vi "Laser handler.vi"(8 "error in (no error)":errorcluster, 11 "Message Queues out":T1) -> (0 "error out":errorcluster, 3 "Message Queue":refnum<queue>)   [LabVIEW 2014]
uses:
  support/Message Queue/All Message Queues.ctl
  support/Message Queue/Message Cluster.ctl
  Engine/Message.ctl
  Teszt/Teszt.ctl
  Teszt/Command.ctl
  Keyence data cluster.ctl
  Keyence Status.ctl
  support/Message Queue/Enqueue Message (Single).vi
  <vilib>/Utility/error.llb/Error Cluster From Error Code.vi
  <vilib>/ErrorRing/Error Ring.xnode
  support/Message Queue/Message Queue.lvlib
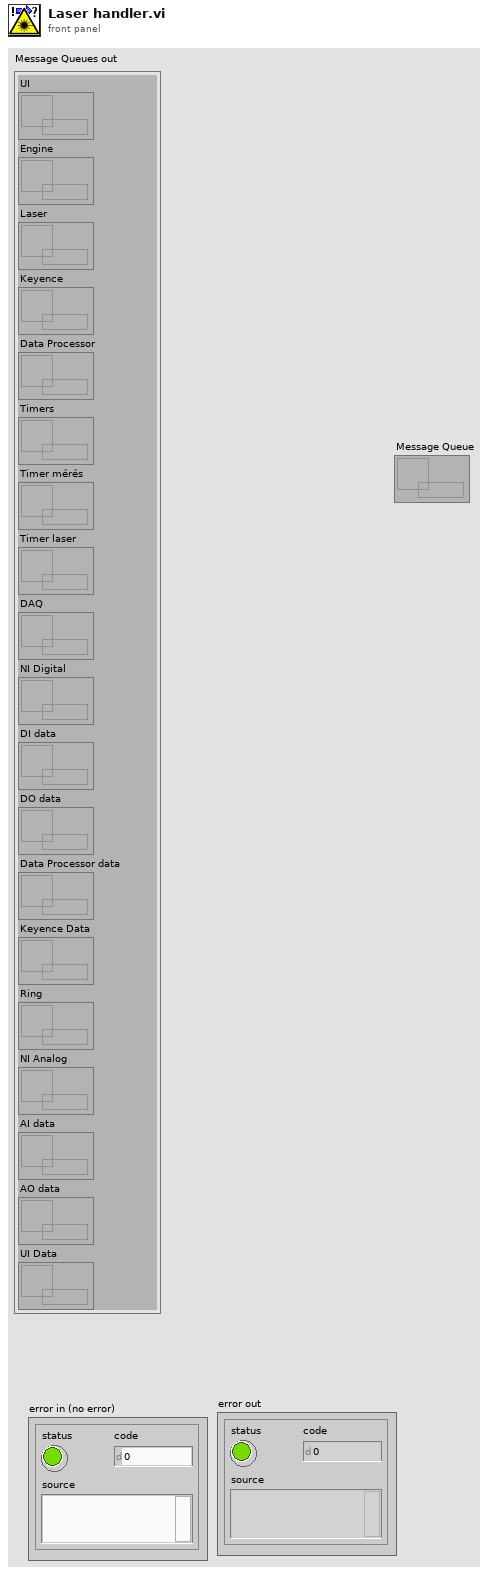
[diagram p1: front panel]
types:
  T1 = typedef "Message Queue.lvlib/All Message Queues.ctl" = cluster{"UI":refnum<queue>, "Engine":refnum<queue>, "Laser":refnum<queue>, "Keyence":refnum<queue>, "Data Processor":refnum<queue>, "Timers":refnum<queue>, "Timer mérés":refnum<queue>, "Timer laser":refnum<queue>, "DAQ":refnum<queue>, "NI Digital":refnum<queue>, "DI data":refnum<queue>, "DO data":refnum<queue>, "Data Processor data":refnum<queue>, "Keyence Data":refnum<queue>, "Ring":refnum<queue>, "NI Analog":refnum<queue>, "AI data":refnum<queue>, "AO data":refnum<queue>, "UI Data":refnum<queue>}
  T2 = typedef "Teszt.ctl" = cluster{"Thread ID":dbl, "Mérésszám":string, "Mérés/Utasítás":string, "Command":T3, "Min":string, "Max":string, "Aktív?":bool, "Log?":bool, "Kiértékelés":bool, "Etalon 1 exp":bool, "Etalon 2 exp":bool, "Etalon 3 exp":bool, "Etalon 4 exp":bool, "Etalon 5 exp":bool}
  T3 = typedef "Command.ctl" = cluster{"Parancs":string, "Paraméter 1":string, "Paraméter 2":string, "Paraméter 3":string, "Paraméter 4":string, "Paraméter 5":string, "Eredmény":string}
  T4 = typedef "Message.ctl" = cluster{"Thread ID":u16, "Callback":string, "Data":variant, "Error":errorcluster}
  T5 = typedef "Keyence data cluster.ctl" = cluster{"Communication Opened":bool, "Status":T6, "IP Address":string, "Laser Disabled":bool}
  T6 = typedef "Keyence Status.ctl" = cluster{"Ready":bool, "Error":bool, "Warning":bool, "Shutter":bool, "Mark Check OK":bool, "Mark Check NG":bool, "Marking Busy":bool, "Program No":u16, "Marking Check Busy":bool, "Marking Completed":bool, "Marking Score":u16, "Marking Error":bool, "Marking Stop":bool, "Program is changing":bool, "Date/Time":timestamp}
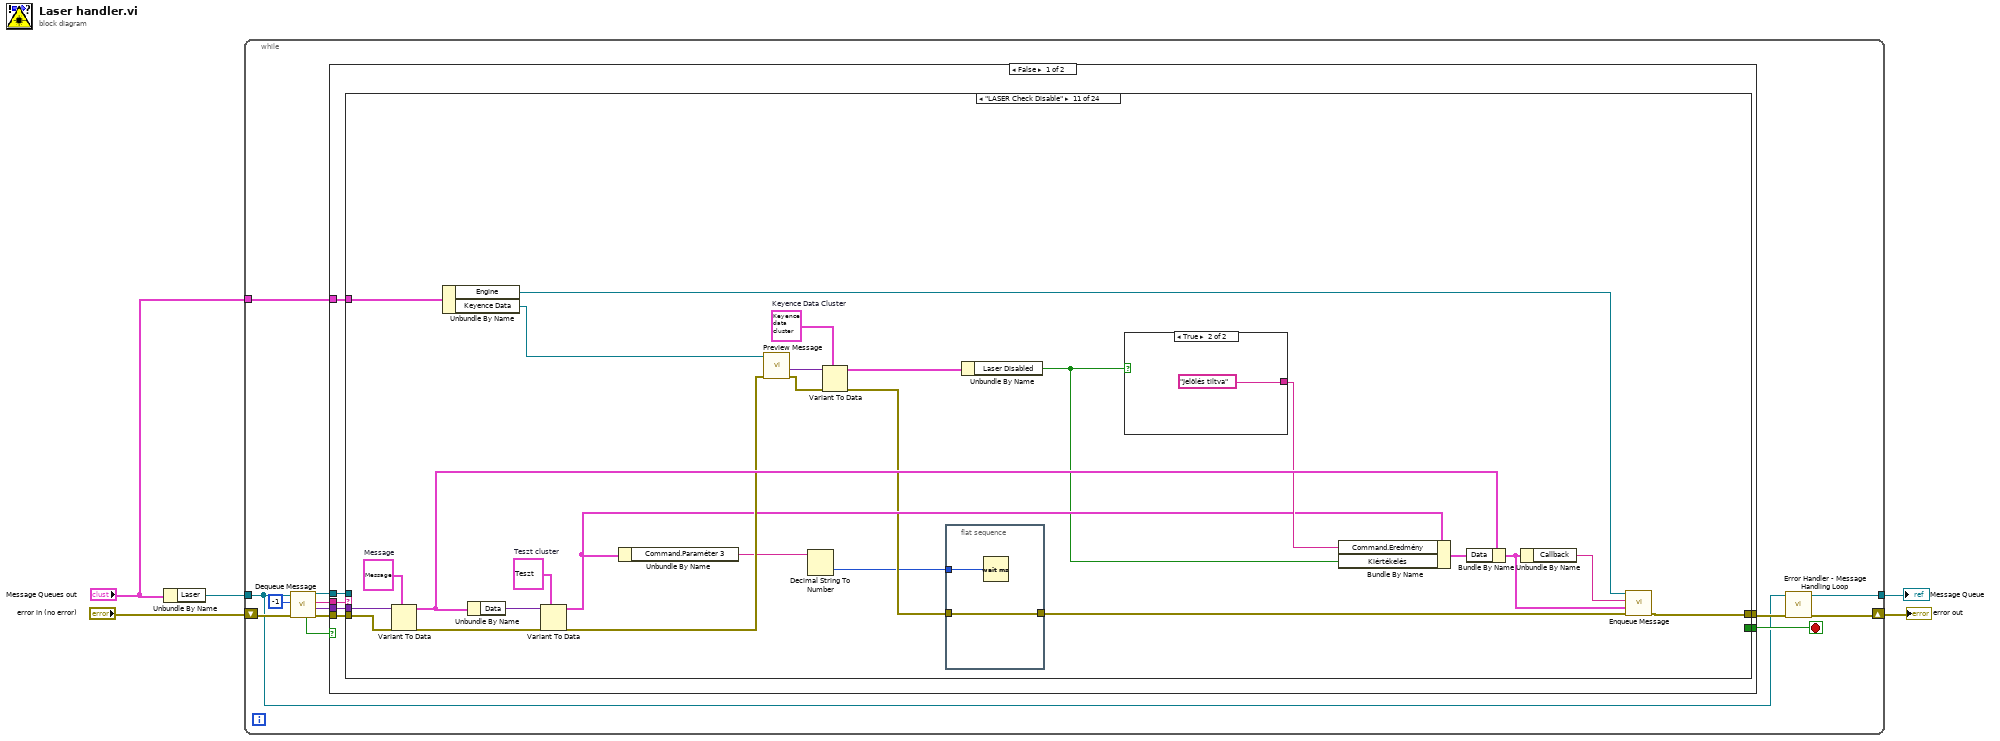
[diagram p0: block diagram]
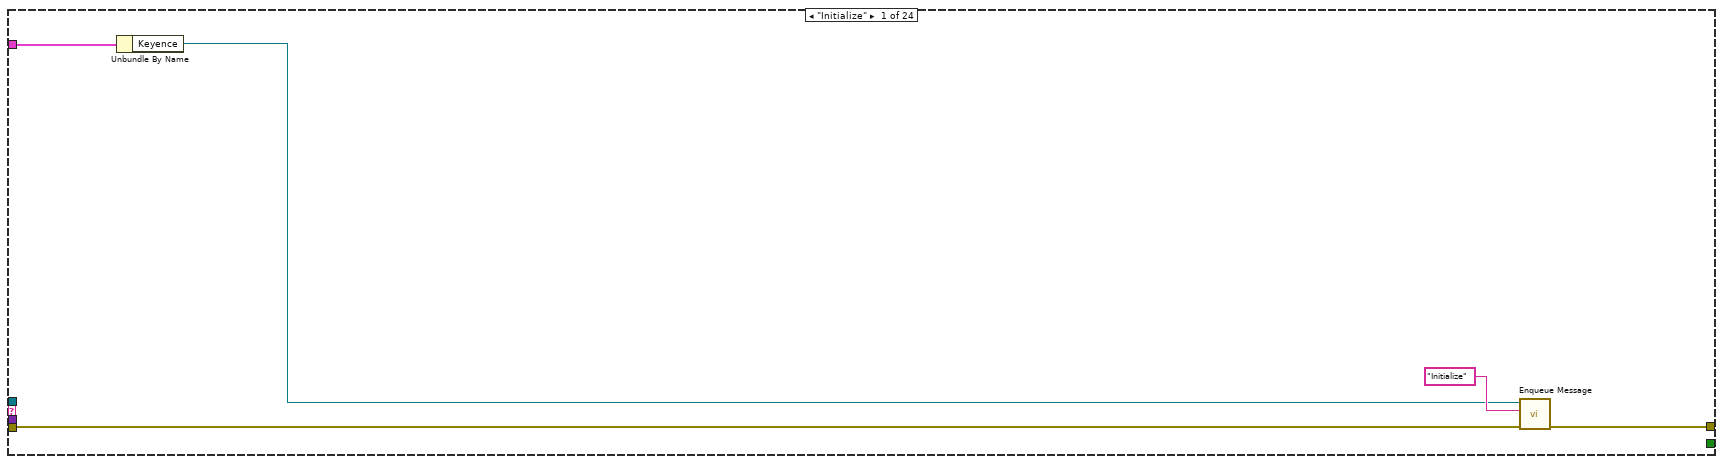
[diagram p2: hidden frame]
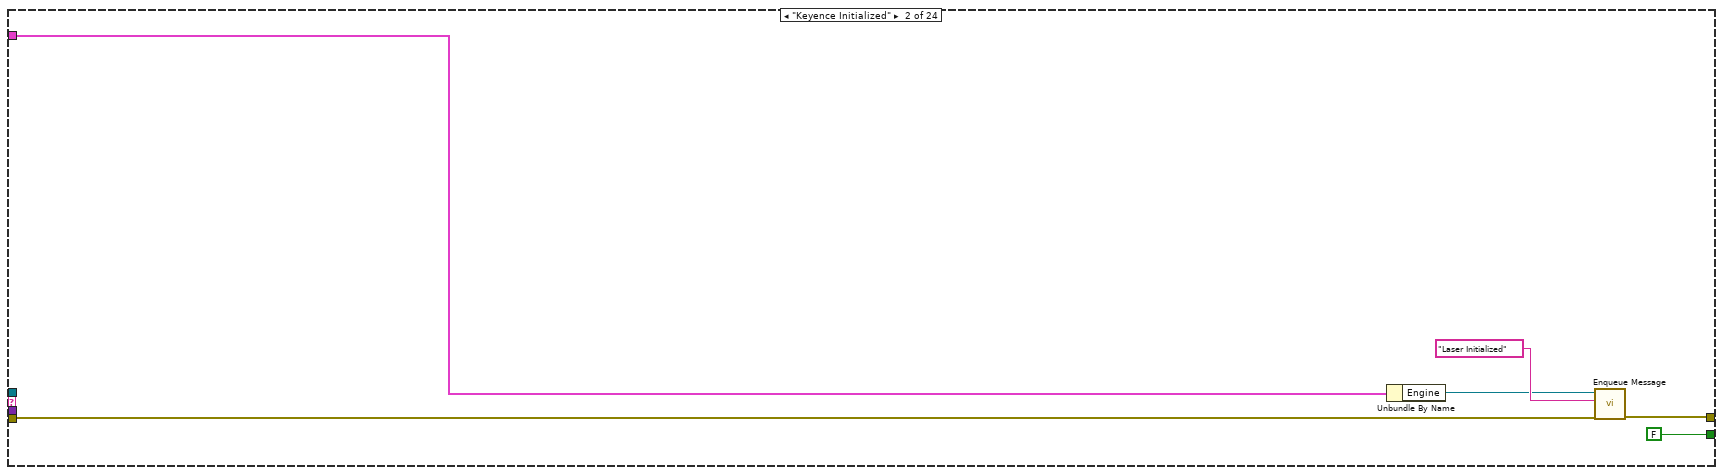
[diagram p3: hidden frame]
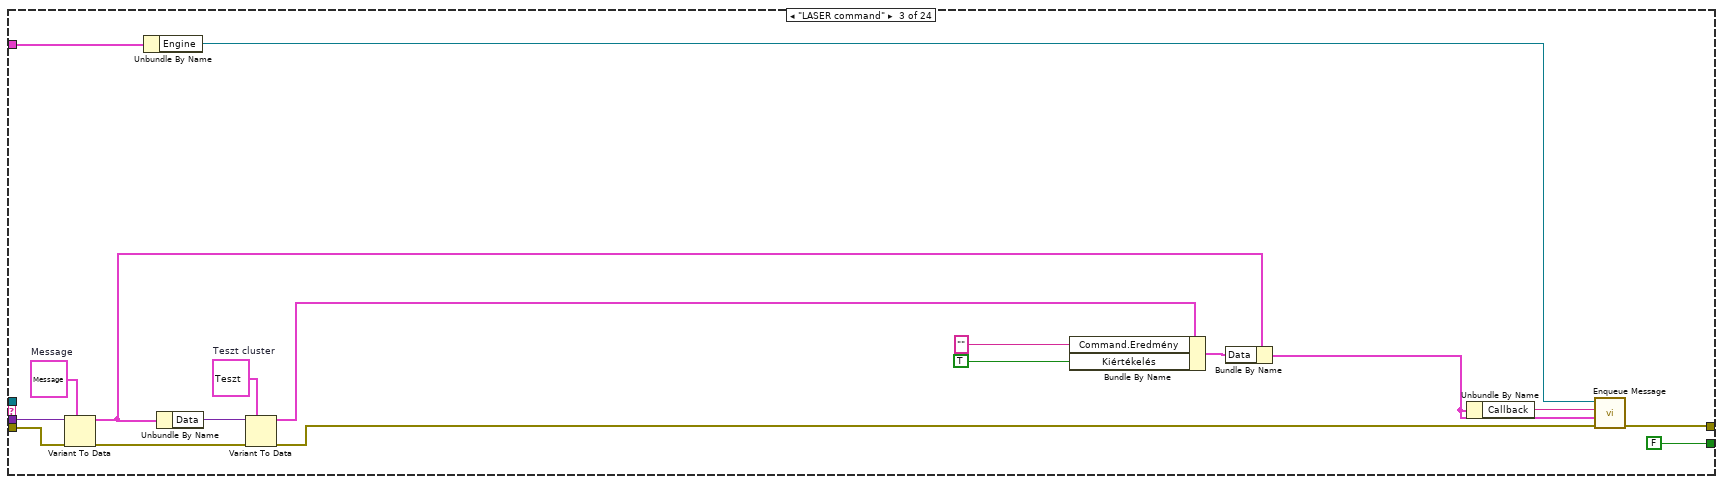
[diagram p4: hidden frame]
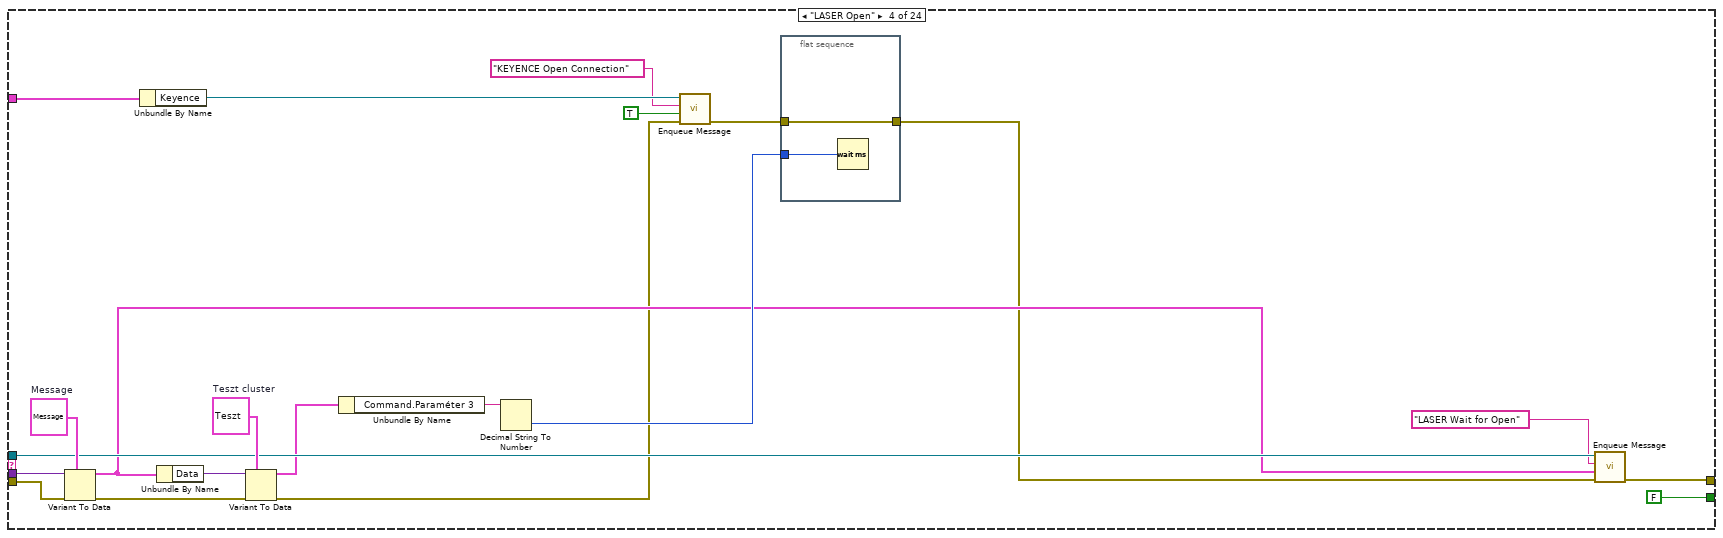
[diagram p5: hidden frame]
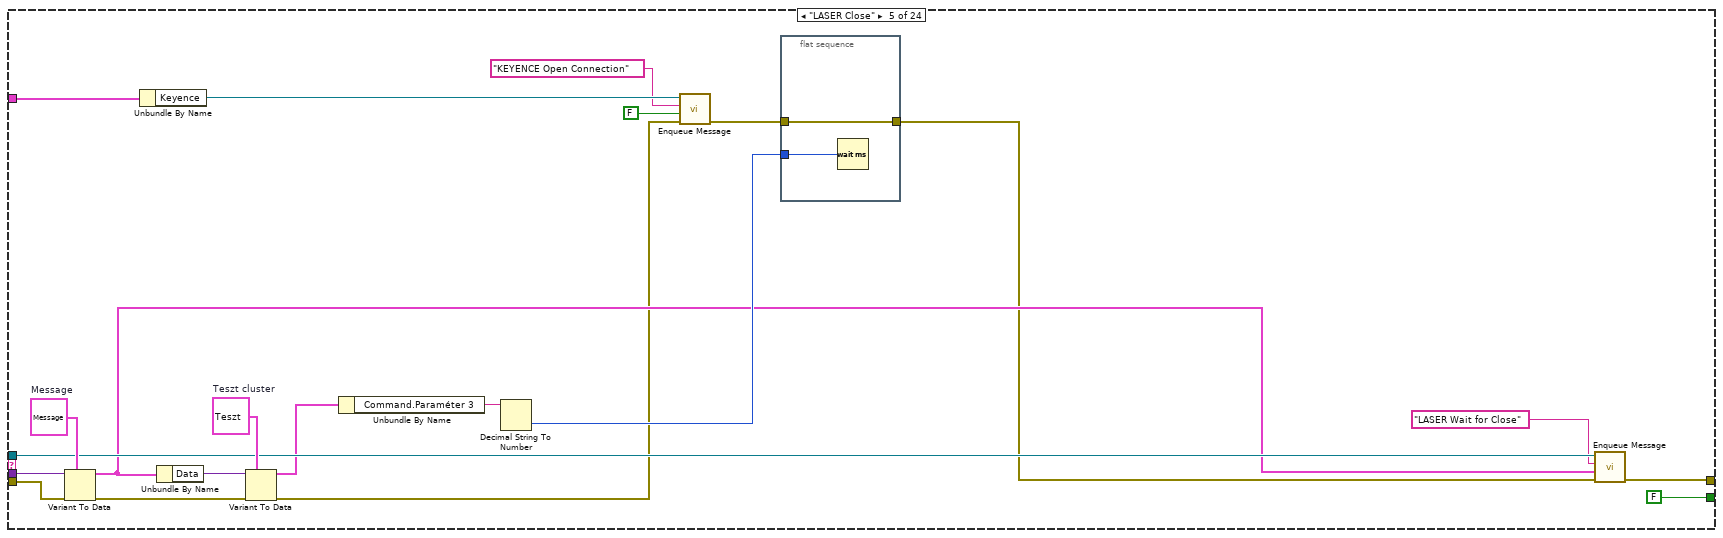
[diagram p6: hidden frame]
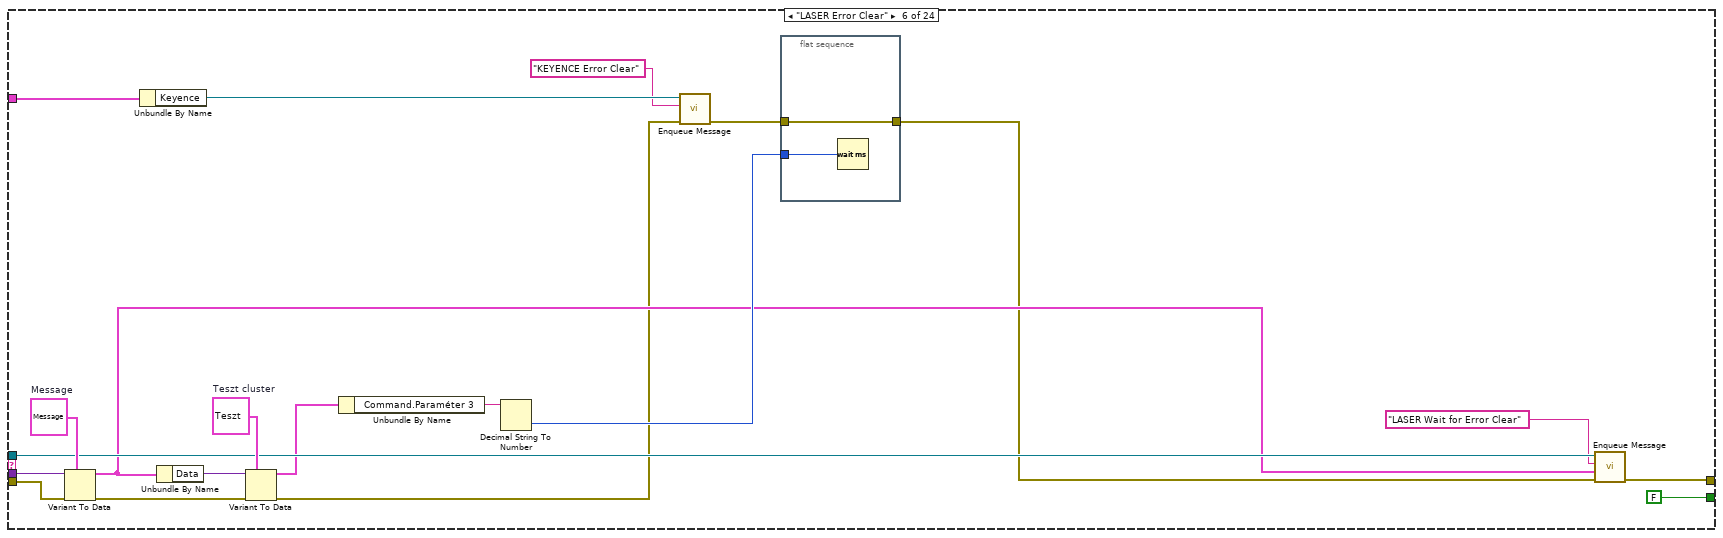
[diagram p7: hidden frame]
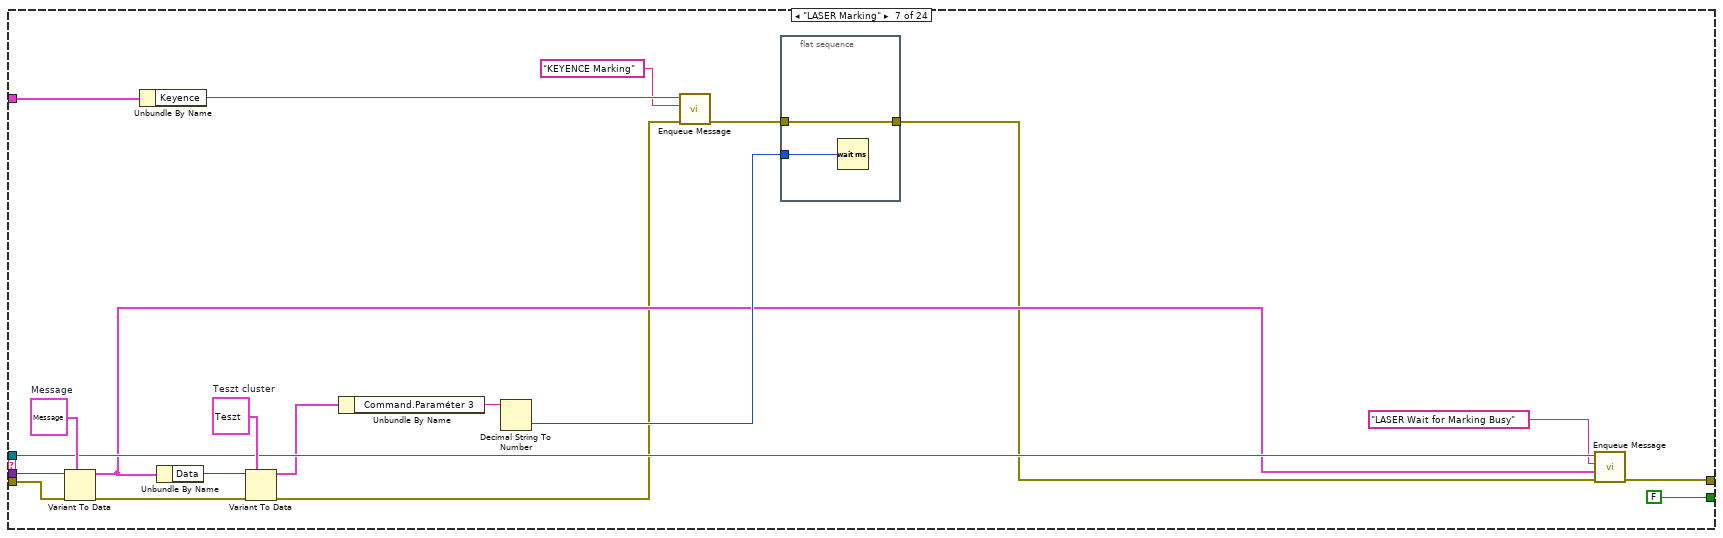
[diagram p8: hidden frame]
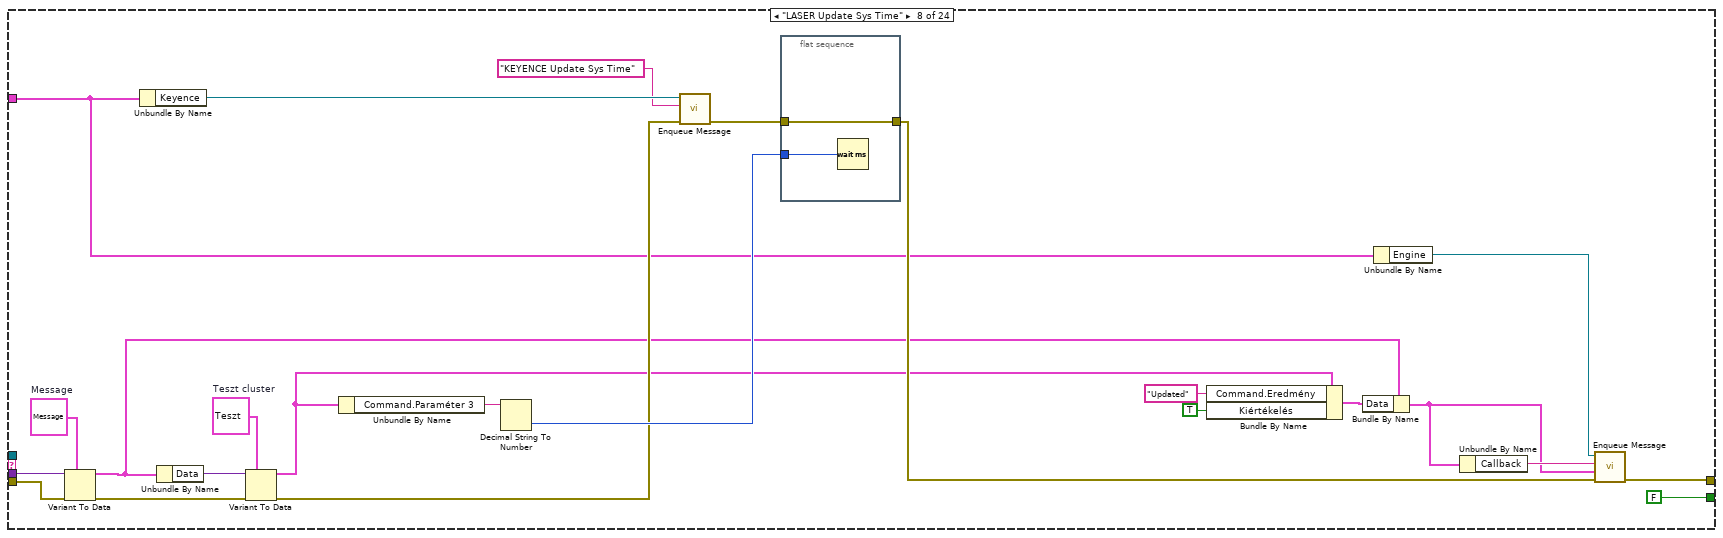
[diagram p9: hidden frame]
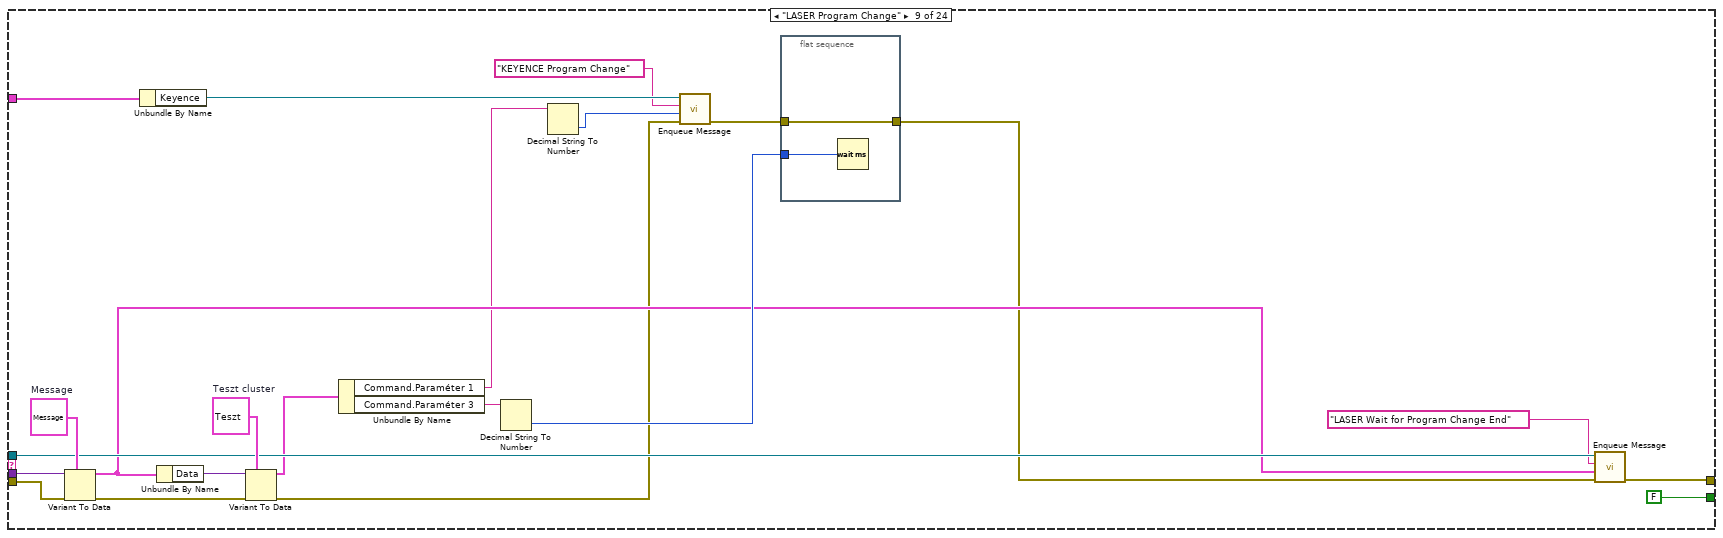
[diagram p10: hidden frame]
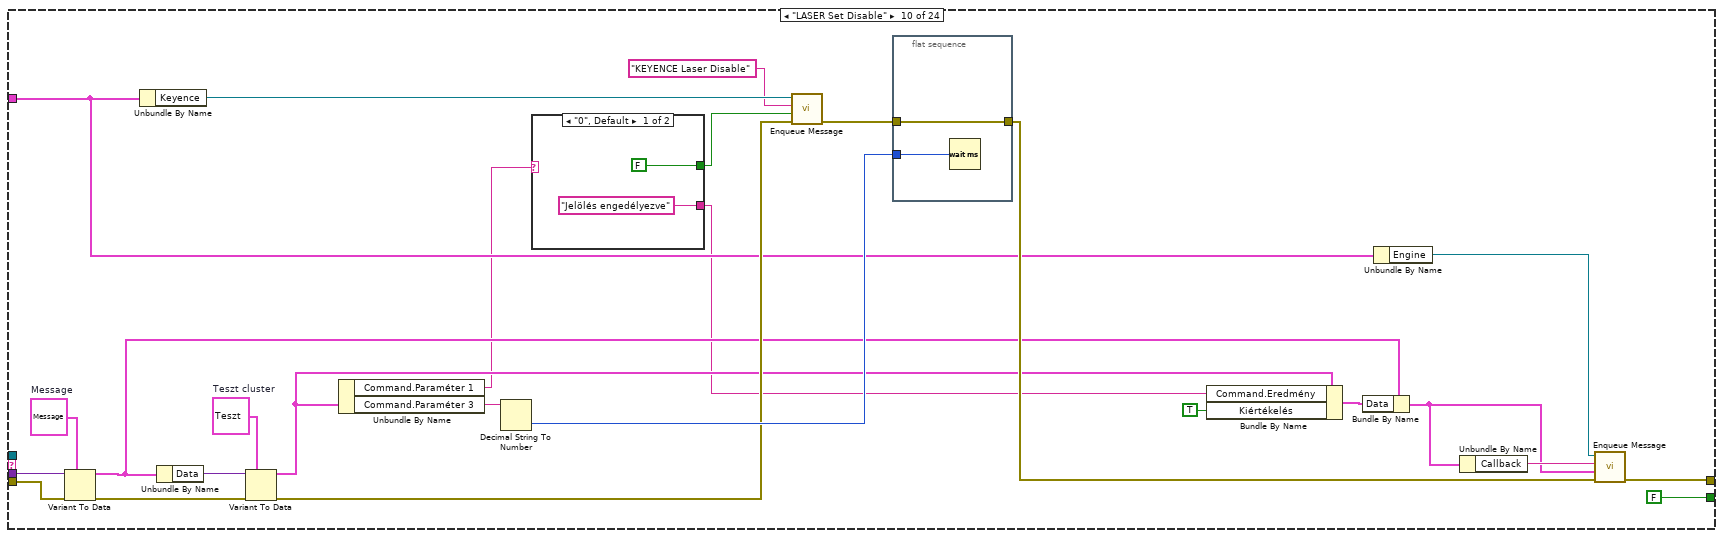
[diagram p11: hidden frame]
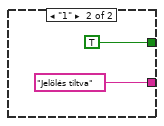
[diagram p12: hidden frame]
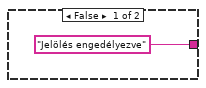
[diagram p13: hidden frame]
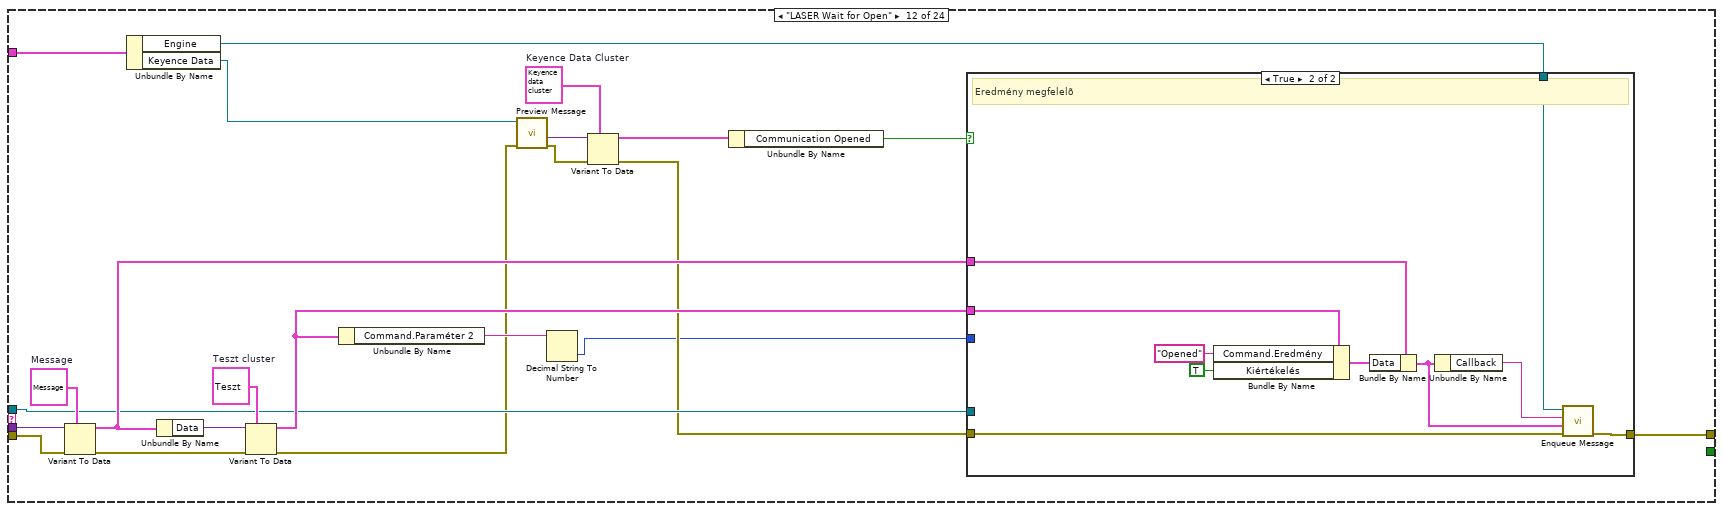
[diagram p14: hidden frame]
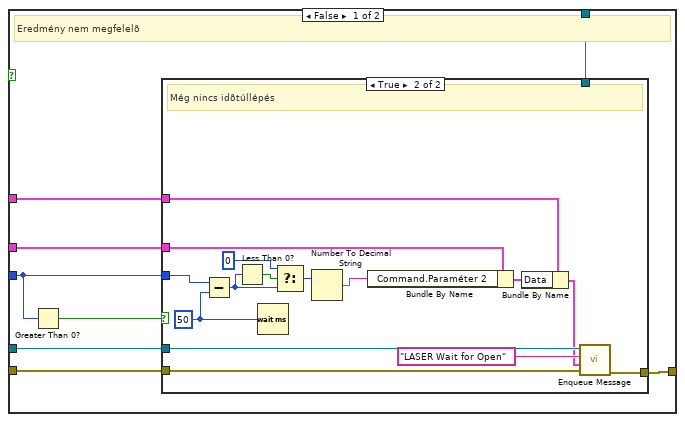
[diagram p15: hidden frame]
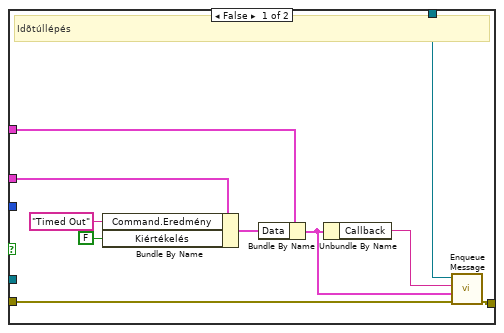
[diagram p16: hidden frame]
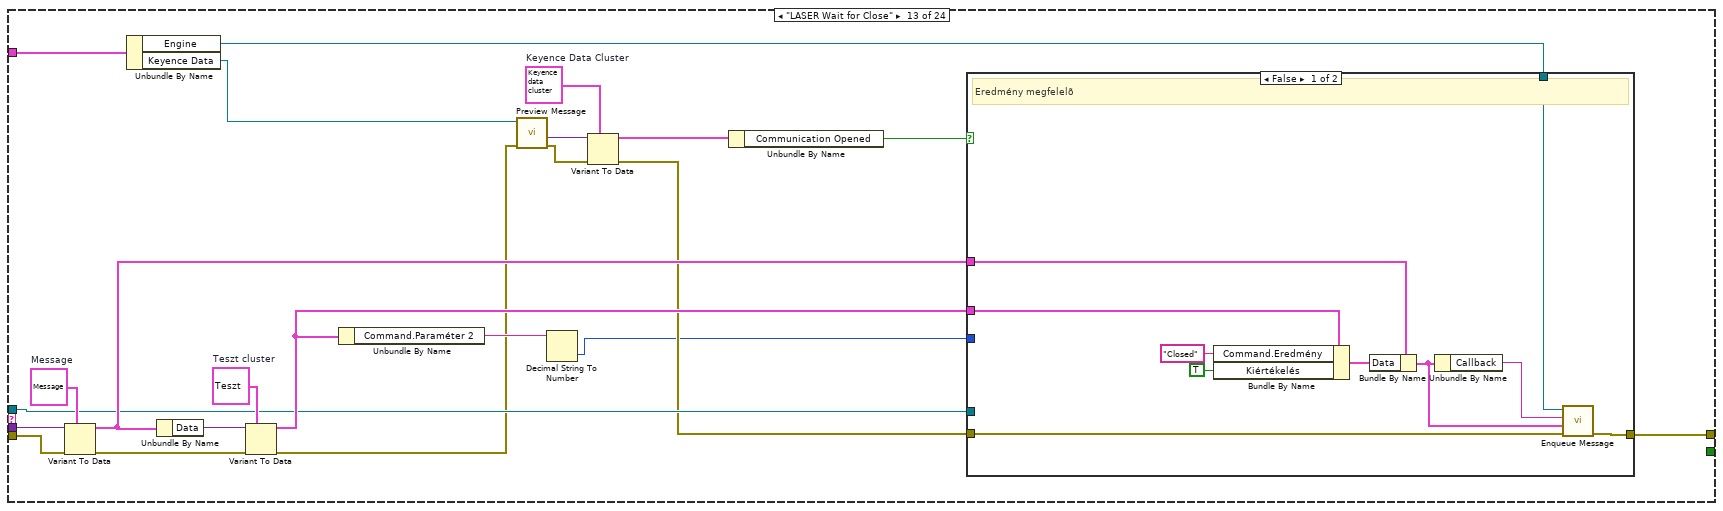
[diagram p17: hidden frame]
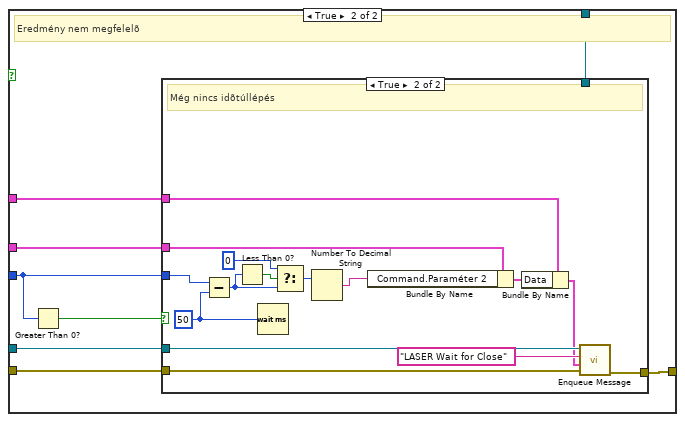
[diagram p18: hidden frame]
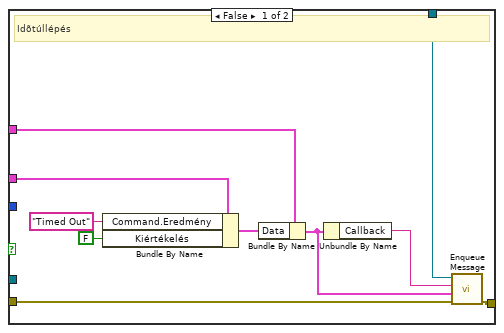
[diagram p19: hidden frame]
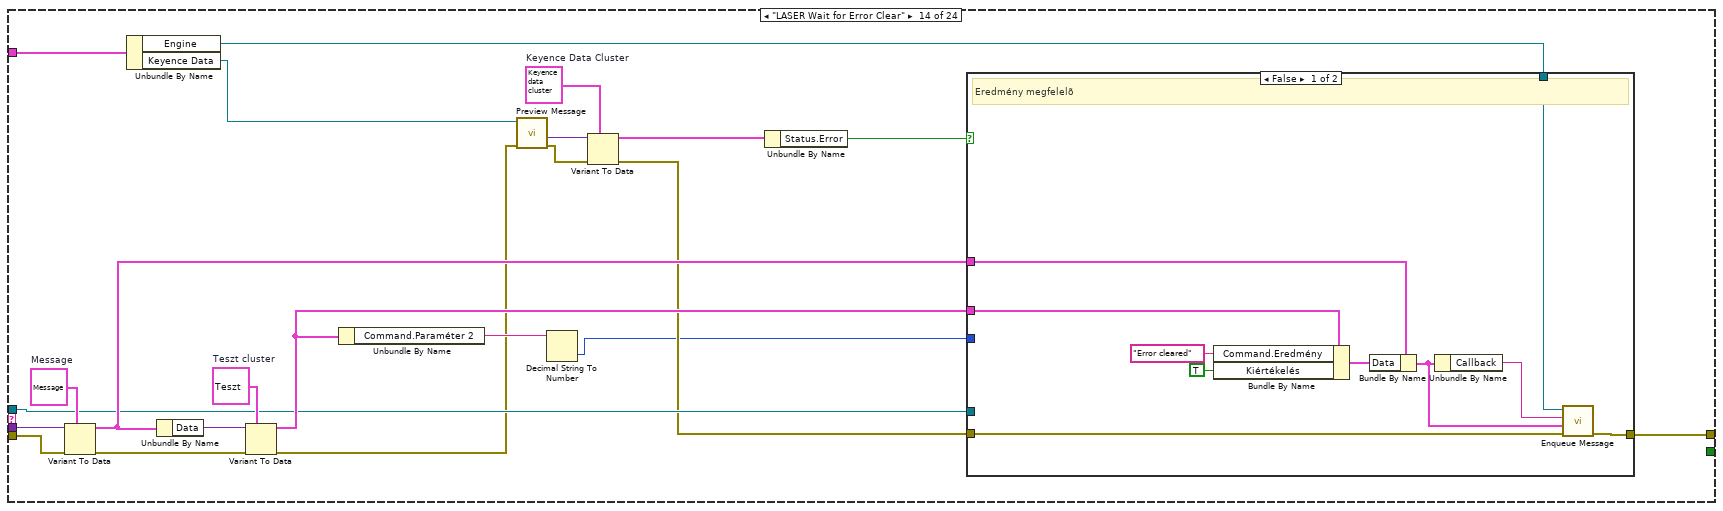
[diagram p20: hidden frame]
diagram:
  n1 = Unbundle By Name("Message Queues out") -> ("Laser"=w2:refnum<queue>)
  n2 = while {
    tunnel: w2 -> [w6]
    shift-right: [w10] -> w5
    shift-left: "error in (no error)" -> [w18]
    tunnel: "Message Queues out" -> [w8]
    tunnel: [w7] -> w1
    stop <- w14 stop-if-true
    n3 = call "Dequeue Message.vi"("error in (no error)"=w18, "timeout in ms (-1)"=-1, "Message Queue"=w6) -> ("error out"=w16:errorcluster, "Message Data"=w11:variant, "Message"=w17:string, "dup Message Queue"=w15:refnum<queue>, "timed out?"=w12:bool)  [unwired: 4 in]
    n4 = case shown="False" w12 {
      tunnel: w17 -> [w25 _]
      tunnel: w16 -> [w24 w804]
      tunnel: w15 -> [w23 _]
      tunnel: [w22 FALSE] -> w14
      tunnel: [w21 w804] -> w9
      tunnel: w11 -> [w20 _]
      tunnel: w8 -> [w19 _]
      frame False {
        n5 = case shown="\"LASER Check Disable\"" w25 {
          selector: w25 -> [_ _ _ _ _ _ _ _ _ _ _ _ _ _ _ _ _ _ _ _ _ _ _ w794]
          tunnel: w24 -> [w28 w31 w46 w68 w91 w113 w135 w163 w185 w215 w245 w271 w336 w401 w466 w529 w589 w651 w720 w773 w774 w788 w791 _]
          tunnel: w23 -> [_ _ _ w66 w89 w111 w133 _ w183 _ _ w265 w330 w395 w460 w523 w583 w645 w714 w772 w777 w787 w793 _]
          tunnel: [w29 w35 w53 w74 w97 w119 w141 w167 w191 w219 w252 w278 w343 w408 w473 w536 w596 w658 w727 w771 w778 w789 w790 w795] -> w21
          tunnel: [_ FALSE FALSE FALSE FALSE FALSE FALSE FALSE FALSE FALSE _ _ _ _ _ _ _ _ _ _ _ _ TRUE FALSE] -> w22
          tunnel: w20 -> [_ _ w45 w67 w90 w112 w134 w162 w184 w214 w244 w270 w335 w400 w465 w528 w588 w650 w719 _ w775 _ _ _]
          tunnel: w19 -> [w27 w32 w51 w73 w96 w118 w140 w146 w190 w199 w250 w276 w341 w406 w471 w534 w594 w656 w725 _ w776 _ _ _]
          frame "Initialize" {
            n6 = Unbundle By Name(w27) -> ("Keyence"=w26:refnum<queue>)
            n7 = call-poly "Enqueue Message.vi"("error in (no error)"=w28, "Message"="Initialize", "Message Queue"=w26) -> ("error out"=w29:errorcluster)  [unwired: 7 in, 1 out]
          }
          frame "Keyence Initialized" {
            n8 = Unbundle By Name(w32) -> ("Engine"=w33:refnum<queue>)
            n9 = call-poly "Enqueue Message.vi"("error in (no error)"=w31, "Message"="Laser Initialized", "Message Queue"=w33) -> ("error out"=w35:errorcluster)  [unwired: 7 in, 1 out]
          }
          frame "LASER command" {
            w47 = T2 {"Thread ID"=0.0, "Mérésszám"="", "Mérés/Utasítás"="", "Command"={"Parancs"="", "Paraméter 1"="", "Paraméter 2"="", "Paraméter 3"="", "Paraméter 4"="", "Paraméter 5"="", "Eredmény"=""}, "Min"="", "Max"="", "Aktív?"=FALSE, "Log?"=FALSE, "Kiértékelés"=FALSE, "Etalon 1 exp"=FALSE, "Etalon 2 exp"=FALSE, "Etalon 3 exp"=FALSE, "Etalon 4 exp"=FALSE, "Etalon 5 exp"=FALSE}  # Teszt cluster
            w50 = T4 {"Thread ID"=0, "Callback"="", "Data"=variant, "Error"={"status"=FALSE, "code"=0, "source"=""}}  # Message
            n10 = Variant To Data(error in=w46, type=w50, Variant=w45) -> (data=w41:T4, error out=w49:errorcluster)
            n11 = Unbundle By Name(w51) -> ("Engine"=w52:refnum<queue>)
            n12 = Unbundle By Name(w41) -> ("Data"=w48:variant)
            n13 = Variant To Data(error in=w49, type=w47, Variant=w48) -> (data=w37:T2, error out=w40:errorcluster)
            n14 = Bundle By Name(cluster=w37, "Command.Eredmény"="", "Kiértékelés"=TRUE) -> (w44:T2)
            n15 = Bundle By Name(cluster=w41, "Data"=w44) -> (w42:T4)
            n16 = Unbundle By Name(w42) -> ("Callback"=w43:string)
            n17 = call-poly "Enqueue Message.vi"("error in (no error)"=w40, "Message Data"=w42, "Message"=w43, "Message Queue"=w52) -> ("error out"=w53:errorcluster)  [unwired: 6 in, 1 out]
          }
          frame "LASER Open" {
            w69 = T2 {"Thread ID"=0.0, "Mérésszám"="", "Mérés/Utasítás"="", "Command"={"Parancs"="", "Paraméter 1"="", "Paraméter 2"="", "Paraméter 3"="", "Paraméter 4"="", "Paraméter 5"="", "Eredmény"=""}, "Min"="", "Max"="", "Aktív?"=FALSE, "Log?"=FALSE, "Kiértékelés"=FALSE, "Etalon 1 exp"=FALSE, "Etalon 2 exp"=FALSE, "Etalon 3 exp"=FALSE, "Etalon 4 exp"=FALSE, "Etalon 5 exp"=FALSE}  # Teszt cluster
            w72 = T4 {"Thread ID"=0, "Callback"="", "Data"=variant, "Error"={"status"=FALSE, "code"=0, "source"=""}}  # Message
            n18 = Variant To Data(error in=w68, type=w72, Variant=w67) -> (data=w58:T4, error out=w71:errorcluster)
            n19 = Unbundle By Name(w73) -> ("Keyence"=w64:refnum<queue>)
            n20 = Unbundle By Name(w58) -> ("Data"=w70:variant)
            n21 = Variant To Data(error in=w71, type=w69, Variant=w70) -> (data=w61:T2, error out=w56:errorcluster)
            n22 = Unbundle By Name(w61) -> ("Command.Paraméter 3"=w60:string)
            n23 = Decimal String To Number(string=w60) -> (number=w59:i32)  [unwired: 2 in, 1 out]
            n24 = call-poly "Enqueue Message.vi"("error in (no error)"=w56, "Message Data"=TRUE, "Message"="KEYENCE Open Connection", "Message Queue"=w64) -> ("error out"=w57:errorcluster)  [unwired: 6 in, 1 out]
            n25 = flat-sequence {
              tunnel: w59 -> [w77]
              tunnel: w57 -> [w76]
              tunnel: [w76] -> w55
              frame #0 {
                n26 = Wait (ms)(milliseconds to wait=w77) -> ()  [unwired: 1 out]
              }
            }
            n27 = call-poly "Enqueue Message.vi"("error in (no error)"=w55, "Message Data"=w58, "Message"="LASER Wait for Open", "Message Queue"=w66) -> ("error out"=w74:errorcluster)  [unwired: 6 in, 1 out]
          }
          frame "LASER Close" {
            w92 = T2 {"Thread ID"=0.0, "Mérésszám"="", "Mérés/Utasítás"="", "Command"={"Parancs"="", "Paraméter 1"="", "Paraméter 2"="", "Paraméter 3"="", "Paraméter 4"="", "Paraméter 5"="", "Eredmény"=""}, "Min"="", "Max"="", "Aktív?"=FALSE, "Log?"=FALSE, "Kiértékelés"=FALSE, "Etalon 1 exp"=FALSE, "Etalon 2 exp"=FALSE, "Etalon 3 exp"=FALSE, "Etalon 4 exp"=FALSE, "Etalon 5 exp"=FALSE}  # Teszt cluster
            w95 = T4 {"Thread ID"=0, "Callback"="", "Data"=variant, "Error"={"status"=FALSE, "code"=0, "source"=""}}  # Message
            n28 = Variant To Data(error in=w91, type=w95, Variant=w90) -> (data=w81:T4, error out=w94:errorcluster)
            n29 = Unbundle By Name(w96) -> ("Keyence"=w87:refnum<queue>)
            n30 = Unbundle By Name(w81) -> ("Data"=w93:variant)
            n31 = Variant To Data(error in=w94, type=w92, Variant=w93) -> (data=w84:T2, error out=w79:errorcluster)
            n32 = Unbundle By Name(w84) -> ("Command.Paraméter 3"=w83:string)
            n33 = Decimal String To Number(string=w83) -> (number=w82:i32)  [unwired: 2 in, 1 out]
            n34 = call-poly "Enqueue Message.vi"("error in (no error)"=w79, "Message Data"=FALSE, "Message"="KEYENCE Open Connection", "Message Queue"=w87) -> ("error out"=w80:errorcluster)  [unwired: 6 in, 1 out]
            n35 = flat-sequence {
              tunnel: w82 -> [w100]
              tunnel: w80 -> [w99]
              tunnel: [w99] -> w78
              frame #0 {
                n36 = Wait (ms)(milliseconds to wait=w100) -> ()  [unwired: 1 out]
              }
            }
            n37 = call-poly "Enqueue Message.vi"("error in (no error)"=w78, "Message Data"=w81, "Message"="LASER Wait for Close", "Message Queue"=w89) -> ("error out"=w97:errorcluster)  [unwired: 6 in, 1 out]
          }
          frame "LASER Error Clear" {
            w114 = T2 {"Thread ID"=0.0, "Mérésszám"="", "Mérés/Utasítás"="", "Command"={"Parancs"="", "Paraméter 1"="", "Paraméter 2"="", "Paraméter 3"="", "Paraméter 4"="", "Paraméter 5"="", "Eredmény"=""}, "Min"="", "Max"="", "Aktív?"=FALSE, "Log?"=FALSE, "Kiértékelés"=FALSE, "Etalon 1 exp"=FALSE, "Etalon 2 exp"=FALSE, "Etalon 3 exp"=FALSE, "Etalon 4 exp"=FALSE, "Etalon 5 exp"=FALSE}  # Teszt cluster
            w117 = T4 {"Thread ID"=0, "Callback"="", "Data"=variant, "Error"={"status"=FALSE, "code"=0, "source"=""}}  # Message
            n38 = Variant To Data(error in=w113, type=w117, Variant=w112) -> (data=w104:T4, error out=w116:errorcluster)
            n39 = Unbundle By Name(w118) -> ("Keyence"=w109:refnum<queue>)
            n40 = Unbundle By Name(w104) -> ("Data"=w115:variant)
            n41 = Variant To Data(error in=w116, type=w114, Variant=w115) -> (data=w107:T2, error out=w102:errorcluster)
            n42 = Unbundle By Name(w107) -> ("Command.Paraméter 3"=w106:string)
            n43 = Decimal String To Number(string=w106) -> (number=w105:i32)  [unwired: 2 in, 1 out]
            n44 = call-poly "Enqueue Message.vi"("error in (no error)"=w102, "Message"="KEYENCE Error Clear", "Message Queue"=w109) -> ("error out"=w103:errorcluster)  [unwired: 7 in, 1 out]
            n45 = flat-sequence {
              tunnel: w105 -> [w122]
              tunnel: w103 -> [w121]
              tunnel: [w121] -> w101
              frame #0 {
                n46 = Wait (ms)(milliseconds to wait=w122) -> ()  [unwired: 1 out]
              }
            }
            n47 = call-poly "Enqueue Message.vi"("error in (no error)"=w101, "Message Data"=w104, "Message"="LASER Wait for Error Clear", "Message Queue"=w111) -> ("error out"=w119:errorcluster)  [unwired: 6 in, 1 out]
          }
          frame "LASER Marking" {
            w136 = T2 {"Thread ID"=0.0, "Mérésszám"="", "Mérés/Utasítás"="", "Command"={"Parancs"="", "Paraméter 1"="", "Paraméter 2"="", "Paraméter 3"="", "Paraméter 4"="", "Paraméter 5"="", "Eredmény"=""}, "Min"="", "Max"="", "Aktív?"=FALSE, "Log?"=FALSE, "Kiértékelés"=FALSE, "Etalon 1 exp"=FALSE, "Etalon 2 exp"=FALSE, "Etalon 3 exp"=FALSE, "Etalon 4 exp"=FALSE, "Etalon 5 exp"=FALSE}  # Teszt cluster
            w139 = T4 {"Thread ID"=0, "Callback"="", "Data"=variant, "Error"={"status"=FALSE, "code"=0, "source"=""}}  # Message
            n48 = Variant To Data(error in=w135, type=w139, Variant=w134) -> (data=w126:T4, error out=w138:errorcluster)
            n49 = Unbundle By Name(w140) -> ("Keyence"=w131:refnum<queue>)
            n50 = Unbundle By Name(w126) -> ("Data"=w137:variant)
            n51 = Variant To Data(error in=w138, type=w136, Variant=w137) -> (data=w129:T2, error out=w124:errorcluster)
            n52 = Unbundle By Name(w129) -> ("Command.Paraméter 3"=w128:string)
            n53 = Decimal String To Number(string=w128) -> (number=w127:i32)  [unwired: 2 in, 1 out]
            n54 = call-poly "Enqueue Message.vi"("error in (no error)"=w124, "Message"="KEYENCE Marking", "Message Queue"=w131) -> ("error out"=w125:errorcluster)  [unwired: 7 in, 1 out]
            n55 = flat-sequence {
              tunnel: w127 -> [w144]
              tunnel: w125 -> [w143]
              tunnel: [w143] -> w123
              frame #0 {
                n56 = Wait (ms)(milliseconds to wait=w144) -> ()  [unwired: 1 out]
              }
            }
            n57 = call-poly "Enqueue Message.vi"("error in (no error)"=w123, "Message Data"=w126, "Message"="LASER Wait for Marking Busy", "Message Queue"=w133) -> ("error out"=w141:errorcluster)  [unwired: 6 in, 1 out]
          }
          frame "LASER Update Sys Time" {
            w164 = T2 {"Thread ID"=0.0, "Mérésszám"="", "Mérés/Utasítás"="", "Command"={"Parancs"="", "Paraméter 1"="", "Paraméter 2"="", "Paraméter 3"="", "Paraméter 4"="", "Paraméter 5"="", "Eredmény"=""}, "Min"="", "Max"="", "Aktív?"=FALSE, "Log?"=FALSE, "Kiértékelés"=FALSE, "Etalon 1 exp"=FALSE, "Etalon 2 exp"=FALSE, "Etalon 3 exp"=FALSE, "Etalon 4 exp"=FALSE, "Etalon 5 exp"=FALSE}  # Teszt cluster
            w148 = T4 {"Thread ID"=0, "Callback"="", "Data"=variant, "Error"={"status"=FALSE, "code"=0, "source"=""}}  # Message
            n58 = Variant To Data(error in=w163, type=w148, Variant=w162) -> (data=w147:T4, error out=w166:errorcluster)
            n59 = Unbundle By Name(w146) -> ("Keyence"=w161:refnum<queue>)
            n60 = Unbundle By Name(w147) -> ("Data"=w165:variant)
            n61 = Variant To Data(error in=w166, type=w164, Variant=w165) -> (data=w149:T2, error out=w156:errorcluster)
            n62 = Unbundle By Name(w149) -> ("Command.Paraméter 3"=w159:string)
            n63 = Decimal String To Number(string=w159) -> (number=w158:i32)  [unwired: 2 in, 1 out]
            n64 = call-poly "Enqueue Message.vi"("error in (no error)"=w156, "Message"="KEYENCE Update Sys Time", "Message Queue"=w161) -> ("error out"=w157:errorcluster)  [unwired: 7 in, 1 out]
            n65 = flat-sequence {
              tunnel: w158 -> [w170]
              tunnel: w157 -> [w169]
              tunnel: [w169] -> w155
              frame #0 {
                n66 = Wait (ms)(milliseconds to wait=w170) -> ()  [unwired: 1 out]
              }
            }
            n67 = Bundle By Name(cluster=w149, "Command.Eredmény"="Updated", "Kiértékelés"=TRUE) -> (w154:T2)
            n68 = Bundle By Name(cluster=w147, "Data"=w154) -> (w150:T4)
            n69 = Unbundle By Name(w146) -> ("Engine"=w145:refnum<queue>)
            n70 = Unbundle By Name(w150) -> ("Callback"=w151:string)
            n71 = call-poly "Enqueue Message.vi"("error in (no error)"=w155, "Message Data"=w150, "Message"=w151, "Message Queue"=w145) -> ("error out"=w167:errorcluster)  [unwired: 6 in, 1 out]
          }
          frame "LASER Program Change" {
            w186 = T2 {"Thread ID"=0.0, "Mérésszám"="", "Mérés/Utasítás"="", "Command"={"Parancs"="", "Paraméter 1"="", "Paraméter 2"="", "Paraméter 3"="", "Paraméter 4"="", "Paraméter 5"="", "Eredmény"=""}, "Min"="", "Max"="", "Aktív?"=FALSE, "Log?"=FALSE, "Kiértékelés"=FALSE, "Etalon 1 exp"=FALSE, "Etalon 2 exp"=FALSE, "Etalon 3 exp"=FALSE, "Etalon 4 exp"=FALSE, "Etalon 5 exp"=FALSE}  # Teszt cluster
            w189 = T4 {"Thread ID"=0, "Callback"="", "Data"=variant, "Error"={"status"=FALSE, "code"=0, "source"=""}}  # Message
            n72 = Variant To Data(error in=w185, type=w189, Variant=w184) -> (data=w176:T4, error out=w188:errorcluster)
            n73 = Unbundle By Name(w190) -> ("Keyence"=w181:refnum<queue>)
            n74 = Unbundle By Name(w176) -> ("Data"=w187:variant)
            n75 = Variant To Data(error in=w188, type=w186, Variant=w187) -> (data=w179:T2, error out=w174:errorcluster)
            n76 = Unbundle By Name(w179) -> ("Command.Paraméter 1"=w172:string, "Command.Paraméter 3"=w178:string)
            n77 = Decimal String To Number(string=w178) -> (number=w177:i32)  [unwired: 2 in, 1 out]
            n78 = Decimal String To Number(string=w172) -> (number=w171:i32)  [unwired: 2 in, 1 out]
            n79 = call-poly "Enqueue Message.vi"("error in (no error)"=w174, "Message Data"=w171, "Message"="KEYENCE Program Change", "Message Queue"=w181) -> ("error out"=w175:errorcluster)  [unwired: 6 in, 1 out]
            n80 = flat-sequence {
              tunnel: w177 -> [w194]
              tunnel: w175 -> [w193]
              tunnel: [w193] -> w173
              frame #0 {
                n81 = Wait (ms)(milliseconds to wait=w194) -> ()  [unwired: 1 out]
              }
            }
            n82 = call-poly "Enqueue Message.vi"("error in (no error)"=w173, "Message Data"=w176, "Message"="LASER Wait for Program Change End", "Message Queue"=w183) -> ("error out"=w191:errorcluster)  [unwired: 6 in, 1 out]
          }
          frame "LASER Set Disable" {
            w216 = T2 {"Thread ID"=0.0, "Mérésszám"="", "Mérés/Utasítás"="", "Command"={"Parancs"="", "Paraméter 1"="", "Paraméter 2"="", "Paraméter 3"="", "Paraméter 4"="", "Paraméter 5"="", "Eredmény"=""}, "Min"="", "Max"="", "Aktív?"=FALSE, "Log?"=FALSE, "Kiértékelés"=FALSE, "Etalon 1 exp"=FALSE, "Etalon 2 exp"=FALSE, "Etalon 3 exp"=FALSE, "Etalon 4 exp"=FALSE, "Etalon 5 exp"=FALSE}  # Teszt cluster
            w201 = T4 {"Thread ID"=0, "Callback"="", "Data"=variant, "Error"={"status"=FALSE, "code"=0, "source"=""}}  # Message
            n83 = Variant To Data(error in=w215, type=w201, Variant=w214) -> (data=w200:T4, error out=w218:errorcluster)
            n84 = Unbundle By Name(w199) -> ("Keyence"=w213:refnum<queue>)
            n85 = Unbundle By Name(w200) -> ("Data"=w217:variant)
            n86 = Variant To Data(error in=w218, type=w216, Variant=w217) -> (data=w202:T2, error out=w208:errorcluster)
            n87 = Unbundle By Name(w202) -> ("Command.Paraméter 1"=w196:string, "Command.Paraméter 3"=w211:string)
            n88 = Decimal String To Number(string=w211) -> (number=w210:i32)  [unwired: 2 in, 1 out]
            n89 = case shown="\"0\", Default" w196 {
              tunnel: [FALSE ("Run") TRUE ("Run")] -> w197
              tunnel: ["Jelölés engedélyezve" "Jelölés tiltva"] -> w195
              frame "0", Default {
              }
              frame "1" {
              }
            }
            n90 = call-poly "Enqueue Message.vi"("error in (no error)"=w208, "Message Data"=w197, "Message"="KEYENCE Laser Disable", "Message Queue"=w213) -> ("error out"=w209:errorcluster)  [unwired: 6 in, 1 out]
            n91 = flat-sequence {
              tunnel: w210 -> [w226]
              tunnel: w209 -> [w225]
              tunnel: [w225] -> w207
              frame #0 {
                n92 = Wait (ms)(milliseconds to wait=w226) -> ()  [unwired: 1 out]
              }
            }
            n93 = Bundle By Name(cluster=w202, "Command.Eredmény"=w195, "Kiértékelés"=TRUE) -> (w206:T2)
            n94 = Bundle By Name(cluster=w200, "Data"=w206) -> (w203:T4)
            n95 = Unbundle By Name(w199) -> ("Engine"=w198:refnum<queue>)
            n96 = Unbundle By Name(w203) -> ("Callback"=w204:string)
            n97 = call-poly "Enqueue Message.vi"("error in (no error)"=w207, "Message Data"=w203, "Message"=w204, "Message Queue"=w198) -> ("error out"=w219:errorcluster)  [unwired: 6 in, 1 out]
          }
          frame "LASER Check Disable" {
            w240 = T5 {"Communication Opened"=FALSE, "Status"={"Ready"=FALSE, "Error"=FALSE, "Warning"=FALSE, "Shutter"=FALSE, "Mark Check OK"=FALSE, "Mark Check NG"=FALSE, "Marking Busy"=FALSE, "Program No"=0, "Marking Check Busy"=FALSE, "Marking Completed"=FALSE, "Marking Score"=0, "Marking Error"=FALSE, "Marking Stop"=FALSE, "Program is changing"=FALSE, "Date/Time"=timestamp(0 s since 1904-01-01)}, "IP Address"="", "Laser Disabled"=FALSE}  # Keyence Data Cluster
            w246 = T2 {"Thread ID"=0.0, "Mérésszám"="", "Mérés/Utasítás"="", "Command"={"Parancs"="", "Paraméter 1"="", "Paraméter 2"="", "Paraméter 3"="", "Paraméter 4"="", "Paraméter 5"="", "Eredmény"=""}, "Min"="", "Max"="", "Aktív?"=FALSE, "Log?"=FALSE, "Kiértékelés"=FALSE, "Etalon 1 exp"=FALSE, "Etalon 2 exp"=FALSE, "Etalon 3 exp"=FALSE, "Etalon 4 exp"=FALSE, "Etalon 5 exp"=FALSE}  # Teszt cluster
            w249 = T4 {"Thread ID"=0, "Callback"="", "Data"=variant, "Error"={"status"=FALSE, "code"=0, "source"=""}}  # Message
            n98 = Variant To Data(error in=w245, type=w249, Variant=w244) -> (data=w243:T4, error out=w248:errorcluster)
            n99 = Unbundle By Name(w250) -> ("Engine"=w251:refnum<queue>, "Keyence Data"=w242:refnum<queue>)
            n100 = Unbundle By Name(w243) -> ("Data"=w247:variant)
            n101 = Variant To Data(error in=w248, type=w246, Variant=w247) -> (data=w232:T2, error out=w237:errorcluster)
            n102 = Unbundle By Name(w232) -> ("Command.Paraméter 3"=w229:string)
            n103 = call "Preview Message.vi"("error in (no error)"=w237, "Message Queue"=w242) -> ("error out"=w238:errorcluster, "Message Data"=w241:variant)  [unwired: 5 in, 3 out]
            n104 = Decimal String To Number(string=w229) -> (number=w228:i32)  [unwired: 2 in, 1 out]
            n105 = Variant To Data(error in=w238, type=w240, Variant=w241) -> (data=w239:T5, error out=w231:errorcluster)
            n106 = flat-sequence {
              tunnel: w228 -> [w254]
              tunnel: w231 -> [w253]
              tunnel: [w253] -> w230
              frame #0 {
                n107 = Wait (ms)(milliseconds to wait=w254) -> ()  [unwired: 1 out]
              }
            }
            n108 = Unbundle By Name(w239) -> ("Laser Disabled"=w227:bool)
            n109 = case shown="True" w227 {
              tunnel: ["Jelölés engedélyezve" ("Command.Eredmény") "Jelölés tiltva" ("Command.Eredmény")] -> w233
              frame False {
              }
              frame True {
              }
            }
            n110 = Bundle By Name(cluster=w232, "Command.Eredmény"=w233, "Kiértékelés"=w227) -> (w235:T2)
            n111 = Bundle By Name(cluster=w243, "Data"=w235) -> (w234:T4)
            n112 = Unbundle By Name(w234) -> ("Callback"=w236:string)
            n113 = call-poly "Enqueue Message.vi"("error in (no error)"=w230, "Message Data"=w234, "Message"=w236, "Message Queue"=w251) -> ("error out"=w252:errorcluster)  [unwired: 6 in, 1 out]
          }
          frame "LASER Wait for Open" {
            w263 = T5 {"Communication Opened"=FALSE, "Status"={"Ready"=FALSE, "Error"=FALSE, "Warning"=FALSE, "Shutter"=FALSE, "Mark Check OK"=FALSE, "Mark Check NG"=FALSE, "Marking Busy"=FALSE, "Program No"=0, "Marking Check Busy"=FALSE, "Marking Completed"=FALSE, "Marking Score"=0, "Marking Error"=FALSE, "Marking Stop"=FALSE, "Program is changing"=FALSE, "Date/Time"=timestamp(0 s since 1904-01-01)}, "IP Address"="", "Laser Disabled"=FALSE}  # Keyence Data Cluster
            w272 = T2 {"Thread ID"=0.0, "Mérésszám"="", "Mérés/Utasítás"="", "Command"={"Parancs"="", "Paraméter 1"="", "Paraméter 2"="", "Paraméter 3"="", "Paraméter 4"="", "Paraméter 5"="", "Eredmény"=""}, "Min"="", "Max"="", "Aktív?"=FALSE, "Log?"=FALSE, "Kiértékelés"=FALSE, "Etalon 1 exp"=FALSE, "Etalon 2 exp"=FALSE, "Etalon 3 exp"=FALSE, "Etalon 4 exp"=FALSE, "Etalon 5 exp"=FALSE}  # Teszt cluster
            w275 = T4 {"Thread ID"=0, "Callback"="", "Data"=variant, "Error"={"status"=FALSE, "code"=0, "source"=""}}  # Message
            n114 = Variant To Data(error in=w271, type=w275, Variant=w270) -> (data=w269:T4, error out=w274:errorcluster)
            n115 = Unbundle By Name(w276) -> ("Engine"=w277:refnum<queue>, "Keyence Data"=w268:refnum<queue>)
            n116 = Unbundle By Name(w269) -> ("Data"=w273:variant)
            n117 = Variant To Data(error in=w274, type=w272, Variant=w273) -> (data=w267:T2, error out=w259:errorcluster)
            n118 = Unbundle By Name(w267) -> ("Command.Paraméter 2"=w266:string)
            n119 = call "Preview Message.vi"("error in (no error)"=w259, "Message Queue"=w268) -> ("error out"=w260:errorcluster, "Message Data"=w264:variant)  [unwired: 5 in, 3 out]
            n120 = Decimal String To Number(string=w266) -> (number=w257:i32)  [unwired: 2 in, 1 out]
            n121 = Variant To Data(error in=w260, type=w263, Variant=w264) -> (data=w262:T5, error out=w258:errorcluster)
            n122 = Unbundle By Name(w262) -> ("Communication Opened"=w261:bool)
            n123 = case shown="True" w261 {
              tunnel: [w286 w321] -> w278
              tunnel: w277 -> [w285 w320]
              tunnel: w269 -> [w284 w316]
              tunnel: w258 -> [w279 w315]
              tunnel: w267 -> [w283 w312]
              tunnel: w257 -> [w281 _]
              tunnel: w265 -> [w280 _]
              frame False {
                # "Eredmény nem megfelelõ"
                n124 = Greater Than 0?(x=w281) -> (x > 0?=w282:bool)
                n125 = case shown="True" w282 {
                  tunnel: [w292 w311] -> w286
                  tunnel: w285 -> [w291 _]
                  tunnel: w284 -> [w290 w307]
                  tunnel: w283 -> [w289 w306]
                  tunnel: w281 -> [_ w304]
                  tunnel: w280 -> [_ w310]
                  tunnel: w279 -> [w287 w297]
                  frame False {
                    # "Idõtúllépés"
                    n126 = Bundle By Name(cluster=w289, "Command.Eredmény"="Timed Out", "Kiértékelés"=FALSE) -> (w293:T2)
                    n127 = Bundle By Name(cluster=w290, "Data"=w293) -> (w288:T4)
                    n128 = Unbundle By Name(w288) -> ("Callback"=w294:string)
                    n129 = call-poly "Enqueue Message.vi"("error in (no error)"=w287, "Message Data"=w288, "Message"=w294, "Message Queue"=w291) -> ("error out"=w292:errorcluster)  [unwired: 6 in, 1 out]
                  }
                  frame True {
                    w303 = 50 ("y")
                    # "Még nincs idõtúllépés"
                    n130 = Subtract(x=w304, y=w303) -> (x-y=w301:i32)
                    n131 = Less Than 0?(x=w301) -> (x < 0?=w302:bool)
                    n132 = Wait (ms)(milliseconds to wait=w303) -> ()  [unwired: 1 out]
                    n133 = Select(t=0, s=w302, f=w301) -> (s? t:f=w299:i32)
                    n134 = Number To Decimal String(number=w299) -> (decimal integer string=w298:string)  [unwired: 1 in]
                    n135 = Bundle By Name(cluster=w306, "Command.Paraméter 2"=w298) -> (w305:T2)
                    n136 = Bundle By Name(cluster=w307, "Data"=w305) -> (w308:T4)
                    n137 = call-poly "Enqueue Message.vi"("error in (no error)"=w297, "Message Data"=w308, "Message"="LASER Wait for Open", "Message Queue"=w310) -> ("error out"=w311:errorcluster)  [unwired: 6 in, 1 out]
                  }
                }
              }
              frame True {
                # "Eredmény megfelelõ"
                n138 = Bundle By Name(cluster=w312, "Command.Eredmény"="Opened", "Kiértékelés"=TRUE) -> (w319:T2)
                n139 = Bundle By Name(cluster=w316, "Data"=w319) -> (w317:T4)
                n140 = Unbundle By Name(w317) -> ("Callback"=w318:string)
                n141 = call-poly "Enqueue Message.vi"("error in (no error)"=w315, "Message Data"=w317, "Message"=w318, "Message Queue"=w320) -> ("error out"=w321:errorcluster)  [unwired: 6 in, 1 out]
              }
            }
          }
          frame "LASER Wait for Close" {
            w328 = T5 {"Communication Opened"=FALSE, "Status"={"Ready"=FALSE, "Error"=FALSE, "Warning"=FALSE, "Shutter"=FALSE, "Mark Check OK"=FALSE, "Mark Check NG"=FALSE, "Marking Busy"=FALSE, "Program No"=0, "Marking Check Busy"=FALSE, "Marking Completed"=FALSE, "Marking Score"=0, "Marking Error"=FALSE, "Marking Stop"=FALSE, "Program is changing"=FALSE, "Date/Time"=timestamp(0 s since 1904-01-01)}, "IP Address"="", "Laser Disabled"=FALSE}  # Keyence Data Cluster
            w337 = T2 {"Thread ID"=0.0, "Mérésszám"="", "Mérés/Utasítás"="", "Command"={"Parancs"="", "Paraméter 1"="", "Paraméter 2"="", "Paraméter 3"="", "Paraméter 4"="", "Paraméter 5"="", "Eredmény"=""}, "Min"="", "Max"="", "Aktív?"=FALSE, "Log?"=FALSE, "Kiértékelés"=FALSE, "Etalon 1 exp"=FALSE, "Etalon 2 exp"=FALSE, "Etalon 3 exp"=FALSE, "Etalon 4 exp"=FALSE, "Etalon 5 exp"=FALSE}  # Teszt cluster
            w340 = T4 {"Thread ID"=0, "Callback"="", "Data"=variant, "Error"={"status"=FALSE, "code"=0, "source"=""}}  # Message
            n142 = Variant To Data(error in=w336, type=w340, Variant=w335) -> (data=w334:T4, error out=w339:errorcluster)
            n143 = Unbundle By Name(w341) -> ("Engine"=w342:refnum<queue>, "Keyence Data"=w333:refnum<queue>)
            n144 = Unbundle By Name(w334) -> ("Data"=w338:variant)
            n145 = Variant To Data(error in=w339, type=w337, Variant=w338) -> (data=w332:T2, error out=w324:errorcluster)
            n146 = Unbundle By Name(w332) -> ("Command.Paraméter 2"=w331:string)
            n147 = call "Preview Message.vi"("error in (no error)"=w324, "Message Queue"=w333) -> ("error out"=w325:errorcluster, "Message Data"=w329:variant)  [unwired: 5 in, 3 out]
            n148 = Decimal String To Number(string=w331) -> (number=w322:i32)  [unwired: 2 in, 1 out]
            n149 = Variant To Data(error in=w325, type=w328, Variant=w329) -> (data=w327:T5, error out=w323:errorcluster)
            n150 = Unbundle By Name(w327) -> ("Communication Opened"=w326:bool)
            n151 = case shown="False" w326 {
              tunnel: [w353 w361] -> w343
              tunnel: w342 -> [w352 w360]
              tunnel: w334 -> [w348 w359]
              tunnel: w323 -> [w347 w354]
              tunnel: w332 -> [w344 w358]
              tunnel: w322 -> [_ w356]
              tunnel: w330 -> [_ w355]
              frame False {
                # "Eredmény megfelelõ"
                n152 = Bundle By Name(cluster=w344, "Command.Eredmény"="Closed", "Kiértékelés"=TRUE) -> (w351:T2)
                n153 = Bundle By Name(cluster=w348, "Data"=w351) -> (w349:T4)
                n154 = Unbundle By Name(w349) -> ("Callback"=w350:string)
                n155 = call-poly "Enqueue Message.vi"("error in (no error)"=w347, "Message Data"=w349, "Message"=w350, "Message Queue"=w352) -> ("error out"=w353:errorcluster)  [unwired: 6 in, 1 out]
              }
              frame True {
                # "Eredmény nem megfelelõ"
                n156 = Greater Than 0?(x=w356) -> (x > 0?=w357:bool)
                n157 = case shown="True" w357 {
                  tunnel: [w367 w386] -> w361
                  tunnel: w360 -> [w366 _]
                  tunnel: w359 -> [w365 w382]
                  tunnel: w358 -> [w364 w381]
                  tunnel: w356 -> [_ w379]
                  tunnel: w355 -> [_ w385]
                  tunnel: w354 -> [w362 w372]
                  frame False {
                    # "Idõtúllépés"
                    n158 = Bundle By Name(cluster=w364, "Command.Eredmény"="Timed Out", "Kiértékelés"=FALSE) -> (w368:T2)
                    n159 = Bundle By Name(cluster=w365, "Data"=w368) -> (w363:T4)
                    n160 = Unbundle By Name(w363) -> ("Callback"=w369:string)
                    n161 = call-poly "Enqueue Message.vi"("error in (no error)"=w362, "Message Data"=w363, "Message"=w369, "Message Queue"=w366) -> ("error out"=w367:errorcluster)  [unwired: 6 in, 1 out]
                  }
                  frame True {
                    w378 = 50 ("y")
                    # "Még nincs idõtúllépés"
                    n162 = Subtract(x=w379, y=w378) -> (x-y=w376:i32)
                    n163 = Less Than 0?(x=w376) -> (x < 0?=w377:bool)
                    n164 = Wait (ms)(milliseconds to wait=w378) -> ()  [unwired: 1 out]
                    n165 = Select(t=0, s=w377, f=w376) -> (s? t:f=w374:i32)
                    n166 = Number To Decimal String(number=w374) -> (decimal integer string=w373:string)  [unwired: 1 in]
                    n167 = Bundle By Name(cluster=w381, "Command.Paraméter 2"=w373) -> (w380:T2)
                    n168 = Bundle By Name(cluster=w382, "Data"=w380) -> (w383:T4)
                    n169 = call-poly "Enqueue Message.vi"("error in (no error)"=w372, "Message Data"=w383, "Message"="LASER Wait for Close", "Message Queue"=w385) -> ("error out"=w386:errorcluster)  [unwired: 6 in, 1 out]
                  }
                }
              }
            }
          }
          frame "LASER Wait for Error Clear" {
            w393 = T5 {"Communication Opened"=FALSE, "Status"={"Ready"=FALSE, "Error"=FALSE, "Warning"=FALSE, "Shutter"=FALSE, "Mark Check OK"=FALSE, "Mark Check NG"=FALSE, "Marking Busy"=FALSE, "Program No"=0, "Marking Check Busy"=FALSE, "Marking Completed"=FALSE, "Marking Score"=0, "Marking Error"=FALSE, "Marking Stop"=FALSE, "Program is changing"=FALSE, "Date/Time"=timestamp(0 s since 1904-01-01)}, "IP Address"="", "Laser Disabled"=FALSE}  # Keyence Data Cluster
            w402 = T2 {"Thread ID"=0.0, "Mérésszám"="", "Mérés/Utasítás"="", "Command"={"Parancs"="", "Paraméter 1"="", "Paraméter 2"="", "Paraméter 3"="", "Paraméter 4"="", "Paraméter 5"="", "Eredmény"=""}, "Min"="", "Max"="", "Aktív?"=FALSE, "Log?"=FALSE, "Kiértékelés"=FALSE, "Etalon 1 exp"=FALSE, "Etalon 2 exp"=FALSE, "Etalon 3 exp"=FALSE, "Etalon 4 exp"=FALSE, "Etalon 5 exp"=FALSE}  # Teszt cluster
            w405 = T4 {"Thread ID"=0, "Callback"="", "Data"=variant, "Error"={"status"=FALSE, "code"=0, "source"=""}}  # Message
            n170 = Variant To Data(error in=w401, type=w405, Variant=w400) -> (data=w399:T4, error out=w404:errorcluster)
            n171 = Unbundle By Name(w406) -> ("Engine"=w407:refnum<queue>, "Keyence Data"=w398:refnum<queue>)
            n172 = Unbundle By Name(w399) -> ("Data"=w403:variant)
            n173 = Variant To Data(error in=w404, type=w402, Variant=w403) -> (data=w397:T2, error out=w390:errorcluster)
            n174 = Unbundle By Name(w397) -> ("Command.Paraméter 2"=w396:string)
            n175 = call "Preview Message.vi"("error in (no error)"=w390, "Message Queue"=w398) -> ("error out"=w391:errorcluster, "Message Data"=w394:variant)  [unwired: 5 in, 3 out]
            n176 = Decimal String To Number(string=w396) -> (number=w388:i32)  [unwired: 2 in, 1 out]
            n177 = Variant To Data(error in=w391, type=w393, Variant=w394) -> (data=w392:T5, error out=w389:errorcluster)
            n178 = Unbundle By Name(w392) -> ("Status.Error"=w387:bool)
            n179 = case shown="False" w387 {
              tunnel: [w418 w426] -> w408
              tunnel: w407 -> [w417 w425]
              tunnel: w399 -> [w413 w424]
              tunnel: w389 -> [w412 w419]
              tunnel: w397 -> [w409 w423]
              tunnel: w388 -> [_ w421]
              tunnel: w395 -> [_ w420]
              frame False {
                # "Eredmény megfelelõ"
                n180 = Bundle By Name(cluster=w409, "Command.Eredmény"="Error cleared", "Kiértékelés"=TRUE) -> (w416:T2)
                n181 = Bundle By Name(cluster=w413, "Data"=w416) -> (w414:T4)
                n182 = Unbundle By Name(w414) -> ("Callback"=w415:string)
                n183 = call-poly "Enqueue Message.vi"("error in (no error)"=w412, "Message Data"=w414, "Message"=w415, "Message Queue"=w417) -> ("error out"=w418:errorcluster)  [unwired: 6 in, 1 out]
              }
              frame True {
                # "Eredmény nem megfelelõ"
                n184 = Greater Than 0?(x=w421) -> (x > 0?=w422:bool)
                n185 = case shown="True" w422 {
                  tunnel: [w432 w451] -> w426
                  tunnel: w425 -> [w431 _]
                  tunnel: w424 -> [w430 w447]
                  tunnel: w423 -> [w429 w446]
                  tunnel: w421 -> [_ w444]
                  tunnel: w420 -> [_ w450]
                  tunnel: w419 -> [w427 w437]
                  frame False {
                    # "Idõtúllépés"
                    n186 = Bundle By Name(cluster=w429, "Command.Eredmény"="Timed Out", "Kiértékelés"=FALSE) -> (w433:T2)
                    n187 = Bundle By Name(cluster=w430, "Data"=w433) -> (w428:T4)
                    n188 = Unbundle By Name(w428) -> ("Callback"=w434:string)
                    n189 = call-poly "Enqueue Message.vi"("error in (no error)"=w427, "Message Data"=w428, "Message"=w434, "Message Queue"=w431) -> ("error out"=w432:errorcluster)  [unwired: 6 in, 1 out]
                  }
                  frame True {
                    w443 = 50 ("y")
                    # "Még nincs idõtúllépés"
                    n190 = Subtract(x=w444, y=w443) -> (x-y=w441:i32)
                    n191 = Less Than 0?(x=w441) -> (x < 0?=w442:bool)
                    n192 = Wait (ms)(milliseconds to wait=w443) -> ()  [unwired: 1 out]
                    n193 = Select(t=0, s=w442, f=w441) -> (s? t:f=w439:i32)
                    n194 = Number To Decimal String(number=w439) -> (decimal integer string=w438:string)  [unwired: 1 in]
                    n195 = Bundle By Name(cluster=w446, "Command.Paraméter 2"=w438) -> (w445:T2)
                    n196 = Bundle By Name(cluster=w447, "Data"=w445) -> (w448:T4)
                    n197 = call-poly "Enqueue Message.vi"("error in (no error)"=w437, "Message Data"=w448, "Message"="LASER Wait for Error Clear", "Message Queue"=w450) -> ("error out"=w451:errorcluster)  [unwired: 6 in, 1 out]
                  }
                }
              }
            }
          }
          frame "LASER Wait for Marking Busy" {
            w458 = T5 {"Communication Opened"=FALSE, "Status"={"Ready"=FALSE, "Error"=FALSE, "Warning"=FALSE, "Shutter"=FALSE, "Mark Check OK"=FALSE, "Mark Check NG"=FALSE, "Marking Busy"=FALSE, "Program No"=0, "Marking Check Busy"=FALSE, "Marking Completed"=FALSE, "Marking Score"=0, "Marking Error"=FALSE, "Marking Stop"=FALSE, "Program is changing"=FALSE, "Date/Time"=timestamp(0 s since 1904-01-01)}, "IP Address"="", "Laser Disabled"=FALSE}  # Keyence Data Cluster
            w467 = T2 {"Thread ID"=0.0, "Mérésszám"="", "Mérés/Utasítás"="", "Command"={"Parancs"="", "Paraméter 1"="", "Paraméter 2"="", "Paraméter 3"="", "Paraméter 4"="", "Paraméter 5"="", "Eredmény"=""}, "Min"="", "Max"="", "Aktív?"=FALSE, "Log?"=FALSE, "Kiértékelés"=FALSE, "Etalon 1 exp"=FALSE, "Etalon 2 exp"=FALSE, "Etalon 3 exp"=FALSE, "Etalon 4 exp"=FALSE, "Etalon 5 exp"=FALSE}  # Teszt cluster
            w470 = T4 {"Thread ID"=0, "Callback"="", "Data"=variant, "Error"={"status"=FALSE, "code"=0, "source"=""}}  # Message
            n198 = Variant To Data(error in=w466, type=w470, Variant=w465) -> (data=w464:T4, error out=w469:errorcluster)
            n199 = Unbundle By Name(w471) -> ("Engine"=w472:refnum<queue>, "Keyence Data"=w463:refnum<queue>)
            n200 = Unbundle By Name(w464) -> ("Data"=w468:variant)
            n201 = Variant To Data(error in=w469, type=w467, Variant=w468) -> (data=w462:T2, error out=w454:errorcluster)
            n202 = Unbundle By Name(w462) -> ("Command.Paraméter 2"=w461:string)
            n203 = call "Preview Message.vi"("error in (no error)"=w454, "Message Queue"=w463) -> ("error out"=w455:errorcluster, "Message Data"=w459:variant)  [unwired: 5 in, 3 out]
            n204 = Decimal String To Number(string=w461) -> (number=w452:i32)  [unwired: 2 in, 1 out]
            n205 = Variant To Data(error in=w455, type=w458, Variant=w459) -> (data=w457:T5, error out=w453:errorcluster)
            n206 = Unbundle By Name(w457) -> ("Status.Marking Busy"=w456:bool)
            n207 = case shown="False" w456 {
              tunnel: [w481 w511] -> w473
              tunnel: w472 -> [w480 _]
              tunnel: w464 -> [w479 w507]
              tunnel: w453 -> [w474 w510]
              tunnel: w462 -> [w478 _]
              tunnel: w452 -> [w476 _]
              tunnel: w460 -> [w475 w509]
              frame False {
                # "Eredmény nem megfelelõ"
                n208 = Greater Than 0?(x=w476) -> (x > 0?=w477:bool)
                n209 = case shown="False" w477 {
                  tunnel: [w487 w506] -> w481
                  tunnel: w480 -> [w486 _]
                  tunnel: w479 -> [w485 w502]
                  tunnel: w478 -> [w484 w501]
                  tunnel: w476 -> [_ w499]
                  tunnel: w475 -> [_ w505]
                  tunnel: w474 -> [w482 w492]
                  frame False {
                    # "Idõtúllépés"
                    n210 = Bundle By Name(cluster=w484, "Command.Eredmény"="Timed Out Marking Busy", "Kiértékelés"=FALSE) -> (w488:T2)
                    n211 = Bundle By Name(cluster=w485, "Data"=w488) -> (w483:T4)
                    n212 = Unbundle By Name(w483) -> ("Callback"=w489:string)
                    n213 = call-poly "Enqueue Message.vi"("error in (no error)"=w482, "Message Data"=w483, "Message"=w489, "Message Queue"=w486) -> ("error out"=w487:errorcluster)  [unwired: 6 in, 1 out]
                  }
                  frame True {
                    w498 = 50 ("y")
                    # "Még nincs idõtúllépés"
                    n214 = Subtract(x=w499, y=w498) -> (x-y=w496:i32)
                    n215 = Less Than 0?(x=w496) -> (x < 0?=w497:bool)
                    n216 = Wait (ms)(milliseconds to wait=w498) -> ()  [unwired: 1 out]
                    n217 = Select(t=0, s=w497, f=w496) -> (s? t:f=w494:i32)
                    n218 = Number To Decimal String(number=w494) -> (decimal integer string=w493:string)  [unwired: 1 in]
                    n219 = Bundle By Name(cluster=w501, "Command.Paraméter 2"=w493) -> (w500:T2)
                    n220 = Bundle By Name(cluster=w502, "Data"=w500) -> (w503:T4)
                    n221 = call-poly "Enqueue Message.vi"("error in (no error)"=w492, "Message Data"=w503, "Message"="LASER Wait for Marking Busy", "Message Queue"=w505) -> ("error out"=w506:errorcluster)  [unwired: 6 in, 1 out]
                  }
                }
              }
              frame True {
                # "Eredmény megfelelõ"
                n222 = call-poly "Enqueue Message.vi"("error in (no error)"=w510, "Message Data"=w507, "Message"="LASER Wait for Marking Completed", "Message Queue"=w509) -> ("error out"=w511:errorcluster)  [unwired: 6 in, 1 out]
              }
            }
          }
          frame "LASER Wait for Marking Completed" {
            w521 = T5 {"Communication Opened"=FALSE, "Status"={"Ready"=FALSE, "Error"=FALSE, "Warning"=FALSE, "Shutter"=FALSE, "Mark Check OK"=FALSE, "Mark Check NG"=FALSE, "Marking Busy"=FALSE, "Program No"=0, "Marking Check Busy"=FALSE, "Marking Completed"=FALSE, "Marking Score"=0, "Marking Error"=FALSE, "Marking Stop"=FALSE, "Program is changing"=FALSE, "Date/Time"=timestamp(0 s since 1904-01-01)}, "IP Address"="", "Laser Disabled"=FALSE}  # Keyence Data Cluster
            w530 = T2 {"Thread ID"=0.0, "Mérésszám"="", "Mérés/Utasítás"="", "Command"={"Parancs"="", "Paraméter 1"="", "Paraméter 2"="", "Paraméter 3"="", "Paraméter 4"="", "Paraméter 5"="", "Eredmény"=""}, "Min"="", "Max"="", "Aktív?"=FALSE, "Log?"=FALSE, "Kiértékelés"=FALSE, "Etalon 1 exp"=FALSE, "Etalon 2 exp"=FALSE, "Etalon 3 exp"=FALSE, "Etalon 4 exp"=FALSE, "Etalon 5 exp"=FALSE}  # Teszt cluster
            w533 = T4 {"Thread ID"=0, "Callback"="", "Data"=variant, "Error"={"status"=FALSE, "code"=0, "source"=""}}  # Message
            n223 = Variant To Data(error in=w529, type=w533, Variant=w528) -> (data=w527:T4, error out=w532:errorcluster)
            n224 = Unbundle By Name(w534) -> ("Engine"=w535:refnum<queue>, "Keyence Data"=w526:refnum<queue>)
            n225 = Unbundle By Name(w527) -> ("Data"=w531:variant)
            n226 = Variant To Data(error in=w532, type=w530, Variant=w531) -> (data=w525:T2, error out=w518:errorcluster)
            n227 = Unbundle By Name(w525) -> ("Command.Paraméter 2"=w524:string)
            n228 = call "Preview Message.vi"("error in (no error)"=w518, "Message Queue"=w526) -> ("error out"=w519:errorcluster, "Message Data"=w522:variant)  [unwired: 5 in, 3 out]
            n229 = Decimal String To Number(string=w524) -> (number=w516:i32)  [unwired: 2 in, 1 out]
            n230 = Variant To Data(error in=w519, type=w521, Variant=w522) -> (data=w520:T5, error out=w517:errorcluster)
            n231 = Unbundle By Name(w520) -> ("Status.Marking Busy"=w512:bool, "Status.Marking Completed"=w514:bool)
            n232 = Not(x=w512) -> (.not. x?=w513:bool)
            n233 = And(x=w513, y=w514) -> (x .and. y?=w515:bool)
            n234 = case shown="True" w515 {
              tunnel: [w544 w574] -> w536
              tunnel: w535 -> [w543 _]
              tunnel: w527 -> [w542 w570]
              tunnel: w517 -> [w537 w573]
              tunnel: w525 -> [w541 _]
              tunnel: w516 -> [w539 _]
              tunnel: w523 -> [w538 w572]
              frame False {
                # "Eredmény nem megfelelõ"
                n235 = Greater Than 0?(x=w539) -> (x > 0?=w540:bool)
                n236 = case shown="False" w540 {
                  tunnel: [w550 w569] -> w544
                  tunnel: w543 -> [w549 _]
                  tunnel: w542 -> [w548 w565]
                  tunnel: w541 -> [w547 w564]
                  tunnel: w539 -> [_ w562]
                  tunnel: w538 -> [_ w568]
                  tunnel: w537 -> [w545 w555]
                  frame False {
                    # "Idõtúllépés"
                    n237 = Bundle By Name(cluster=w547, "Command.Eredmény"="Timed Out Marking Completed", "Kiértékelés"=FALSE) -> (w551:T2)
                    n238 = Bundle By Name(cluster=w548, "Data"=w551) -> (w546:T4)
                    n239 = Unbundle By Name(w546) -> ("Callback"=w552:string)
                    n240 = call-poly "Enqueue Message.vi"("error in (no error)"=w545, "Message Data"=w546, "Message"=w552, "Message Queue"=w549) -> ("error out"=w550:errorcluster)  [unwired: 6 in, 1 out]
                  }
                  frame True {
                    w561 = 50 ("y")
                    # "Még nincs idõtúllépés"
                    n241 = Subtract(x=w562, y=w561) -> (x-y=w559:i32)
                    n242 = Less Than 0?(x=w559) -> (x < 0?=w560:bool)
                    n243 = Wait (ms)(milliseconds to wait=w561) -> ()  [unwired: 1 out]
                    n244 = Select(t=0, s=w560, f=w559) -> (s? t:f=w557:i32)
                    n245 = Number To Decimal String(number=w557) -> (decimal integer string=w556:string)  [unwired: 1 in]
                    n246 = Bundle By Name(cluster=w564, "Command.Paraméter 2"=w556) -> (w563:T2)
                    n247 = Bundle By Name(cluster=w565, "Data"=w563) -> (w566:T4)
                    n248 = call-poly "Enqueue Message.vi"("error in (no error)"=w555, "Message Data"=w566, "Message"="LASER Wait for Marking Completed", "Message Queue"=w568) -> ("error out"=w569:errorcluster)  [unwired: 6 in, 1 out]
                  }
                }
              }
              frame True {
                # "Eredmény megfelelõ"
                n249 = call-poly "Enqueue Message.vi"("error in (no error)"=w573, "Message Data"=w570, "Message"="LASER Wait for Check", "Message Queue"=w572) -> ("error out"=w574:errorcluster)  [unwired: 6 in, 1 out]
              }
            }
          }
          frame "LASER Wait for Check" {
            w581 = T5 {"Communication Opened"=FALSE, "Status"={"Ready"=FALSE, "Error"=FALSE, "Warning"=FALSE, "Shutter"=FALSE, "Mark Check OK"=FALSE, "Mark Check NG"=FALSE, "Marking Busy"=FALSE, "Program No"=0, "Marking Check Busy"=FALSE, "Marking Completed"=FALSE, "Marking Score"=0, "Marking Error"=FALSE, "Marking Stop"=FALSE, "Program is changing"=FALSE, "Date/Time"=timestamp(0 s since 1904-01-01)}, "IP Address"="", "Laser Disabled"=FALSE}  # Keyence Data Cluster
            w590 = T2 {"Thread ID"=0.0, "Mérésszám"="", "Mérés/Utasítás"="", "Command"={"Parancs"="", "Paraméter 1"="", "Paraméter 2"="", "Paraméter 3"="", "Paraméter 4"="", "Paraméter 5"="", "Eredmény"=""}, "Min"="", "Max"="", "Aktív?"=FALSE, "Log?"=FALSE, "Kiértékelés"=FALSE, "Etalon 1 exp"=FALSE, "Etalon 2 exp"=FALSE, "Etalon 3 exp"=FALSE, "Etalon 4 exp"=FALSE, "Etalon 5 exp"=FALSE}  # Teszt cluster
            w593 = T4 {"Thread ID"=0, "Callback"="", "Data"=variant, "Error"={"status"=FALSE, "code"=0, "source"=""}}  # Message
            n250 = Variant To Data(error in=w589, type=w593, Variant=w588) -> (data=w587:T4, error out=w592:errorcluster)
            n251 = Unbundle By Name(w594) -> ("Engine"=w595:refnum<queue>, "Keyence Data"=w586:refnum<queue>)
            n252 = Unbundle By Name(w587) -> ("Data"=w591:variant)
            n253 = Variant To Data(error in=w592, type=w590, Variant=w591) -> (data=w585:T2, error out=w578:errorcluster)
            n254 = Unbundle By Name(w585) -> ("Command.Paraméter 2"=w584:string)
            n255 = call "Preview Message.vi"("error in (no error)"=w578, "Message Queue"=w586) -> ("error out"=w579:errorcluster, "Message Data"=w582:variant)  [unwired: 5 in, 3 out]
            n256 = Decimal String To Number(string=w584) -> (number=w576:i32)  [unwired: 2 in, 1 out]
            n257 = Variant To Data(error in=w579, type=w581, Variant=w582) -> (data=w580:T5, error out=w577:errorcluster)
            n258 = Unbundle By Name(w580) -> ("Status.Marking Check Busy"=w575:bool)
            n259 = case shown="False" w575 {
              tunnel: [w604 w634] -> w596
              tunnel: w595 -> [w603 _]
              tunnel: w587 -> [w602 w630]
              tunnel: w577 -> [w597 w633]
              tunnel: w585 -> [w601 _]
              tunnel: w576 -> [w599 _]
              tunnel: w583 -> [w598 w632]
              frame False {
                # "Eredmény nem megfelelõ"
                n260 = Greater Than 0?(x=w599) -> (x > 0?=w600:bool)
                n261 = case shown="False" w600 {
                  tunnel: [w610 w629] -> w604
                  tunnel: w603 -> [w609 _]
                  tunnel: w602 -> [w608 w625]
                  tunnel: w601 -> [w607 w624]
                  tunnel: w599 -> [_ w622]
                  tunnel: w598 -> [_ w628]
                  tunnel: w597 -> [w605 w615]
                  frame False {
                    # "Idõtúllépés"
                    n262 = Bundle By Name(cluster=w607, "Command.Eredmény"="Timed Out Check Busy", "Kiértékelés"=FALSE) -> (w611:T2)
                    n263 = Bundle By Name(cluster=w608, "Data"=w611) -> (w606:T4)
                    n264 = Unbundle By Name(w606) -> ("Callback"=w612:string)
                    n265 = call-poly "Enqueue Message.vi"("error in (no error)"=w605, "Message Data"=w606, "Message"=w612, "Message Queue"=w609) -> ("error out"=w610:errorcluster)  [unwired: 6 in, 1 out]
                  }
                  frame True {
                    w621 = 50 ("y")
                    # "Még nincs idõtúllépés"
                    n266 = Subtract(x=w622, y=w621) -> (x-y=w619:i32)
                    n267 = Less Than 0?(x=w619) -> (x < 0?=w620:bool)
                    n268 = Wait (ms)(milliseconds to wait=w621) -> ()  [unwired: 1 out]
                    n269 = Select(t=0, s=w620, f=w619) -> (s? t:f=w617:i32)
                    n270 = Number To Decimal String(number=w617) -> (decimal integer string=w616:string)  [unwired: 1 in]
                    n271 = Bundle By Name(cluster=w624, "Command.Paraméter 2"=w616) -> (w623:T2)
                    n272 = Bundle By Name(cluster=w625, "Data"=w623) -> (w626:T4)
                    n273 = call-poly "Enqueue Message.vi"("error in (no error)"=w615, "Message Data"=w626, "Message"="LASER Wait for Check", "Message Queue"=w628) -> ("error out"=w629:errorcluster)  [unwired: 6 in, 1 out]
                  }
                }
              }
              frame True {
                # "Eredmény megfelelõ"
                n274 = call-poly "Enqueue Message.vi"("error in (no error)"=w633, "Message Data"=w630, "Message"="LASER Wait for Check End", "Message Queue"=w632) -> ("error out"=w634:errorcluster)  [unwired: 6 in, 1 out]
              }
            }
          }
          frame "LASER Wait for Check End" {
            w643 = T5 {"Communication Opened"=FALSE, "Status"={"Ready"=FALSE, "Error"=FALSE, "Warning"=FALSE, "Shutter"=FALSE, "Mark Check OK"=FALSE, "Mark Check NG"=FALSE, "Marking Busy"=FALSE, "Program No"=0, "Marking Check Busy"=FALSE, "Marking Completed"=FALSE, "Marking Score"=0, "Marking Error"=FALSE, "Marking Stop"=FALSE, "Program is changing"=FALSE, "Date/Time"=timestamp(0 s since 1904-01-01)}, "IP Address"="", "Laser Disabled"=FALSE}  # Keyence Data Cluster
            w652 = T2 {"Thread ID"=0.0, "Mérésszám"="", "Mérés/Utasítás"="", "Command"={"Parancs"="", "Paraméter 1"="", "Paraméter 2"="", "Paraméter 3"="", "Paraméter 4"="", "Paraméter 5"="", "Eredmény"=""}, "Min"="", "Max"="", "Aktív?"=FALSE, "Log?"=FALSE, "Kiértékelés"=FALSE, "Etalon 1 exp"=FALSE, "Etalon 2 exp"=FALSE, "Etalon 3 exp"=FALSE, "Etalon 4 exp"=FALSE, "Etalon 5 exp"=FALSE}  # Teszt cluster
            w655 = T4 {"Thread ID"=0, "Callback"="", "Data"=variant, "Error"={"status"=FALSE, "code"=0, "source"=""}}  # Message
            n275 = Variant To Data(error in=w651, type=w655, Variant=w650) -> (data=w649:T4, error out=w654:errorcluster)
            n276 = Unbundle By Name(w656) -> ("Engine"=w657:refnum<queue>, "Keyence Data"=w648:refnum<queue>)
            n277 = Unbundle By Name(w649) -> ("Data"=w653:variant)
            n278 = Variant To Data(error in=w654, type=w652, Variant=w653) -> (data=w647:T2, error out=w640:errorcluster)
            n279 = Unbundle By Name(w647) -> ("Command.Paraméter 2"=w646:string)
            n280 = call "Preview Message.vi"("error in (no error)"=w640, "Message Queue"=w648) -> ("error out"=w641:errorcluster, "Message Data"=w644:variant)  [unwired: 5 in, 3 out]
            n281 = Decimal String To Number(string=w646) -> (number=w638:i32)  [unwired: 2 in, 1 out]
            n282 = Variant To Data(error in=w641, type=w643, Variant=w644) -> (data=w642:T5, error out=w639:errorcluster)
            n283 = Unbundle By Name(w642) -> ("Status.Marking Check Busy"=w637:bool, "Status.Mark Check OK"=w636:bool, "Status.Marking Score"=w635:u16)
            n284 = case shown="False" w637 {
              tunnel: [w669 w677] -> w658
              tunnel: w657 -> [w659 w676]
              tunnel: w649 -> [w668 w675]
              tunnel: w639 -> [w667 w670]
              tunnel: w647 -> [w665 w674]
              tunnel: w638 -> [_ w672]
              tunnel: w645 -> [_ w671]
              tunnel: w636 -> [w664 _]
              tunnel: w635 -> [w661 _]
              frame False {
                # "Eredmény megfelelõ"
                n285 = Number To Decimal String(number=w661) -> (decimal integer string=w660:string)  [unwired: 1 in]
                n286 = Bundle By Name(cluster=w665, "Command.Eredmény"=w660, "Kiértékelés"=w664) -> (w666:T2)
                n287 = Bundle By Name(cluster=w668, "Data"=w666) -> (w663:T4)
                n288 = Unbundle By Name(w663) -> ("Callback"=w662:string)
                n289 = call-poly "Enqueue Message.vi"("error in (no error)"=w667, "Message Data"=w663, "Message"=w662, "Message Queue"=w659) -> ("error out"=w669:errorcluster)  [unwired: 6 in, 1 out]
              }
              frame True {
                # "Eredmény nem megfelelõ"
                n290 = Greater Than 0?(x=w672) -> (x > 0?=w673:bool)
                n291 = case shown="False" w673 {
                  tunnel: [w683 w702] -> w677
                  tunnel: w676 -> [w682 _]
                  tunnel: w675 -> [w681 w698]
                  tunnel: w674 -> [w680 w697]
                  tunnel: w672 -> [_ w695]
                  tunnel: w671 -> [_ w701]
                  tunnel: w670 -> [w678 w688]
                  frame False {
                    # "Idõtúllépés"
                    n292 = Bundle By Name(cluster=w680, "Command.Eredmény"="Timed Out Check End", "Kiértékelés"=FALSE) -> (w684:T2)
                    n293 = Bundle By Name(cluster=w681, "Data"=w684) -> (w679:T4)
                    n294 = Unbundle By Name(w679) -> ("Callback"=w685:string)
                    n295 = call-poly "Enqueue Message.vi"("error in (no error)"=w678, "Message Data"=w679, "Message"=w685, "Message Queue"=w682) -> ("error out"=w683:errorcluster)  [unwired: 6 in, 1 out]
                  }
                  frame True {
                    w694 = 50 ("y")
                    # "Még nincs idõtúllépés"
                    n296 = Subtract(x=w695, y=w694) -> (x-y=w692:i32)
                    n297 = Less Than 0?(x=w692) -> (x < 0?=w693:bool)
                    n298 = Wait (ms)(milliseconds to wait=w694) -> ()  [unwired: 1 out]
                    n299 = Select(t=0, s=w693, f=w692) -> (s? t:f=w690:i32)
                    n300 = Number To Decimal String(number=w690) -> (decimal integer string=w689:string)  [unwired: 1 in]
                    n301 = Bundle By Name(cluster=w697, "Command.Paraméter 2"=w689) -> (w696:T2)
                    n302 = Bundle By Name(cluster=w698, "Data"=w696) -> (w699:T4)
                    n303 = call-poly "Enqueue Message.vi"("error in (no error)"=w688, "Message Data"=w699, "Message"="LASER Wait for Check End", "Message Queue"=w701) -> ("error out"=w702:errorcluster)  [unwired: 6 in, 1 out]
                  }
                }
              }
            }
          }
          frame "LASER Wait for Program Change End" {
            w712 = T5 {"Communication Opened"=FALSE, "Status"={"Ready"=FALSE, "Error"=FALSE, "Warning"=FALSE, "Shutter"=FALSE, "Mark Check OK"=FALSE, "Mark Check NG"=FALSE, "Marking Busy"=FALSE, "Program No"=0, "Marking Check Busy"=FALSE, "Marking Completed"=FALSE, "Marking Score"=0, "Marking Error"=FALSE, "Marking Stop"=FALSE, "Program is changing"=FALSE, "Date/Time"=timestamp(0 s since 1904-01-01)}, "IP Address"="", "Laser Disabled"=FALSE}  # Keyence Data Cluster
            w721 = T2 {"Thread ID"=0.0, "Mérésszám"="", "Mérés/Utasítás"="", "Command"={"Parancs"="", "Paraméter 1"="", "Paraméter 2"="", "Paraméter 3"="", "Paraméter 4"="", "Paraméter 5"="", "Eredmény"=""}, "Min"="", "Max"="", "Aktív?"=FALSE, "Log?"=FALSE, "Kiértékelés"=FALSE, "Etalon 1 exp"=FALSE, "Etalon 2 exp"=FALSE, "Etalon 3 exp"=FALSE, "Etalon 4 exp"=FALSE, "Etalon 5 exp"=FALSE}  # Teszt cluster
            w724 = T4 {"Thread ID"=0, "Callback"="", "Data"=variant, "Error"={"status"=FALSE, "code"=0, "source"=""}}  # Message
            n304 = Variant To Data(error in=w720, type=w724, Variant=w719) -> (data=w718:T4, error out=w723:errorcluster)
            n305 = Unbundle By Name(w725) -> ("Engine"=w726:refnum<queue>, "Keyence Data"=w717:refnum<queue>)
            n306 = Unbundle By Name(w718) -> ("Data"=w722:variant)
            n307 = Variant To Data(error in=w723, type=w721, Variant=w722) -> (data=w716:T2, error out=w709:errorcluster)
            n308 = Unbundle By Name(w716) -> ("Command.Paraméter 1"=w704:string, "Command.Paraméter 2"=w715:string)
            n309 = call "Preview Message.vi"("error in (no error)"=w709, "Message Queue"=w717) -> ("error out"=w710:errorcluster, "Message Data"=w713:variant)  [unwired: 5 in, 3 out]
            n310 = Decimal String To Number(string=w715) -> (number=w707:i32)  [unwired: 2 in, 1 out]
            n311 = Variant To Data(error in=w710, type=w712, Variant=w713) -> (data=w711:T5, error out=w708:errorcluster)
            n312 = Unbundle By Name(w711) -> ("Status.Program No"=w705:u16)
            n313 = Decimal String To Number(string=w704) -> (number=w703:i32)  [unwired: 2 in, 1 out]
            n314 = Equal?(x=w705, y=w703) -> (x = y?=w706:bool)
            n315 = case shown="True" w706 {
              tunnel: [w735 w770] -> w727
              tunnel: w726 -> [w734 w761]
              tunnel: w718 -> [w733 w769]
              tunnel: w708 -> [w728 w768]
              tunnel: w716 -> [w732 w766]
              tunnel: w707 -> [w730 _]
              tunnel: w714 -> [w729 _]
              frame False {
                # "Eredmény nem megfelelõ"
                n316 = Greater Than 0?(x=w730) -> (x > 0?=w731:bool)
                n317 = case shown="False" w731 {
                  tunnel: [w741 w760] -> w735
                  tunnel: w734 -> [w740 _]
                  tunnel: w733 -> [w739 w756]
                  tunnel: w732 -> [w738 w755]
                  tunnel: w730 -> [_ w753]
                  tunnel: w729 -> [_ w759]
                  tunnel: w728 -> [w736 w746]
                  frame False {
                    # "Idõtúllépés"
                    n318 = Bundle By Name(cluster=w738, "Command.Eredmény"="Timed Out Program Change End", "Kiértékelés"=FALSE) -> (w742:T2)
                    n319 = Bundle By Name(cluster=w739, "Data"=w742) -> (w737:T4)
                    n320 = Unbundle By Name(w737) -> ("Callback"=w743:string)
                    n321 = call-poly "Enqueue Message.vi"("error in (no error)"=w736, "Message Data"=w737, "Message"=w743, "Message Queue"=w740) -> ("error out"=w741:errorcluster)  [unwired: 6 in, 1 out]
                  }
                  frame True {
                    w752 = 50 ("y")
                    # "Még nincs idõtúllépés"
                    n322 = Subtract(x=w753, y=w752) -> (x-y=w750:i32)
                    n323 = Less Than 0?(x=w750) -> (x < 0?=w751:bool)
                    n324 = Wait (ms)(milliseconds to wait=w752) -> ()  [unwired: 1 out]
                    n325 = Select(t=0, s=w751, f=w750) -> (s? t:f=w748:i32)
                    n326 = Number To Decimal String(number=w748) -> (decimal integer string=w747:string)  [unwired: 1 in]
                    n327 = Bundle By Name(cluster=w755, "Command.Paraméter 2"=w747) -> (w754:T2)
                    n328 = Bundle By Name(cluster=w756, "Data"=w754) -> (w757:T4)
                    n329 = call-poly "Enqueue Message.vi"("error in (no error)"=w746, "Message Data"=w757, "Message"="LASER Wait for Program Change End", "Message Queue"=w759) -> ("error out"=w760:errorcluster)  [unwired: 6 in, 1 out]
                  }
                }
              }
              frame True {
                # "Eredmény megfelelõ"
                n330 = Bundle By Name(cluster=w766, "Command.Eredmény"="Program changed", "Kiértékelés"=TRUE) -> (w767:T2)
                n331 = Bundle By Name(cluster=w769, "Data"=w767) -> (w765:T4)
                n332 = Unbundle By Name(w765) -> ("Callback"=w764:string)
                n333 = call-poly "Enqueue Message.vi"("error in (no error)"=w768, "Message Data"=w765, "Message"=w764, "Message Queue"=w761) -> ("error out"=w770:errorcluster)  [unwired: 6 in, 1 out]
              }
            }
          }
          frame "Abort" {
            n334 = Flush Queue(queue=w772, error in (no error)=w773) -> (error out=w771:errorcluster)  [unwired: 2 out]
          }
          frame "Error" {
            n335 = Unbundle By Name(w776) -> ("UI"=w781:refnum<queue>)
            n336 = call-poly "Enqueue Message.vi"("error in (no error)"=w774, "Message Data"=w775, "Message"="Error", "Message Queue"=w781) -> ("error out"=w783:errorcluster)  [unwired: 6 in, 1 out]
            n337 = call-poly "Enqueue Message.vi"("Priority Message? (F)"=TRUE, "error in (no error)"=w774, "Message"="Initiate Stop", "Message Queue"=w777) -> ("error out"=w782:errorcluster)  [unwired: 6 in, 1 out]
            n338 = Merge Errors(w783, w782) -> (w778:errorcluster)
          }
          frame "Initiate Stop" {
            n339 = call-poly "Enqueue Message.vi"("Priority Message? (F)"=TRUE, "error in (no error)"=w788, "Message"="Program Stop", "Message Queue"=w787) -> ("error out"=w789:errorcluster)  [unwired: 6 in, 1 out]
          }
          frame "Program Stop" {
            n340 = Flush Queue(queue=w793, error in (no error)=w791) -> (error out=w790:errorcluster)  [unwired: 2 out]
          }
          frame Default {
            n341 = xnode "Error Ring"("parameter 0"=w794) -> ("error out"=w795:errorcluster)
          }
        }
      }
      frame True {
      }
    }
    n342 = call "Error Handler - Message Handling Loop.vi"("error in (no error)"=w9, "Message Queue"=w6) -> ("dup error in"=w10:errorcluster, "dup Message Queue"=w7:refnum<queue>)  [unwired: 8 in]
  }
  "error out" <- w5
  "Message Queue" <- w1
